vi "Autonomous Independent.vi"() -> ()   [LabVIEW 2019]
doc: "This VI is called when autonomous begins, and will automatically be terminated when autonomous ends. You can carry out timed or sensor driven robot movement independently without needing to return to the caller."
uses:
  <vilib>/Rock Robotics/WPI/ThirdParty/Phoenix-LabVIEW/Motor Controller/Controls/CTRE_Phoenix_MotorControl_ControlMode.ctl
  <vilib>/Rock Robotics/Network Tables/NT Read String.vi
  GlobalRefnum.vi
  Global Vars.vi
  <vilib>/Rock Robotics/WPI/ThirdParty/Phoenix-LabVIEW/Motor Controller/Get/CTRE_Phoenix_MotorController_GetSelectedSensorData.vi
  <vilib>/Rock Robotics/WPI/Utilities/WPI_GetSetVariantRefNum.vi
  Joystick_Buttons.vi
  <vilib>/Rock Robotics/Network Tables/NT Write Number.vi
  <vilib>/Rock Robotics/Network Tables/NT Write Numeric Array.vi
panel:
  in  "Travel Distance (In) 6":i32=223200
  out "Left Pos (In) 7":i32
  out "Right Pos (In) 7":i32
  in  "DriveK 7":dbl=0.01 min=0.0 max=1.0 step=0.05
  in  "MaxDrive Fast 5":dbl(slide)=0.7518248175182481 min=0.0 max=1.0 step=0.01 scale=0.0..1.0
  in  "DriveDeadband 7":dbl=100.0
  in  "MaxDrive Slow 4":dbl(slide)=0.49635036496350365 min=0.0 max=1.0 step=0.01 scale=0.0..1.0
  out "Left Pos (In) 6":i32
  out "Right Pos (In) 6":i32
  in  "DriveK 6":dbl=0.01 min=0.0 max=1.0 step=0.05
  in  "MaxDrive Fast 4":dbl(slide)=0.7518248175182481 min=0.0 max=1.0 step=0.01 scale=0.0..1.0
  in  "DriveDeadband 6":dbl=100.0
  in  "MaxDrive Slow 3":dbl(slide)=0.49635036496350365 min=0.0 max=1.0 step=0.01 scale=0.0..1.0
  in  "Reverse? 6":bool=TRUE
  in  "Tab Control":T1(tab)
  in  "Travel Distance (In)":dbl=36.0
  out "Left Pos (In)":dbl
  out "Right Pos (In)":dbl
  in  "Reverse?":bool
  in  "Output":dbl(slide)=-0.5 scale=0.0..1.0
  in  "Travel Distance (In) 3":i32=30000
  in  "Reverse? 3":bool
  out "Left Pos (In) 3":i32
  out "Right Pos (In) 3":i32
  in  "DriveK 2":dbl=0.01 min=0.0 max=1.0 step=0.05
  in  "DriveDeadband 2":dbl=100.0
  in  "MaxDrive 2":dbl(slide)=0.6824817518248175 min=0.0 max=1.0 step=0.01 scale=0.0..1.0
  in  "Reverse? 4":bool=TRUE
  out "Right Pos (In) 4":i32
  out "Left Pos (In) 4":i32
  in  "Travel Distance (In) 4":i32=223200
  in  "DriveDeadband 3":dbl=100.0
  in  "DriveK 3":dbl=0.01 min=0.0 max=1.0 step=0.05
  in  "MaxDrive Fast":dbl(slide)=0.7518248175182481 min=0.0 max=1.0 step=0.01 scale=0.0..1.0
  in  "MaxDrive Slow":dbl(slide)=0.49635036496350365 min=0.0 max=1.0 step=0.01 scale=0.0..1.0
  in  "DriveDeadband 4":dbl=100.0
  in  "DriveDeadband 5":dbl=100.0
  out "Right Pos (In) 5":i32
  out "Left Pos (In) 5":i32
  in  "DriveK 4":dbl=0.01 min=0.0 max=1.0 step=0.05
  in  "DriveK 5":dbl=0.01 min=0.0 max=1.0 step=0.05
  in  "Reverse? 5":bool=TRUE
  in  "Travel Distance (In) 5":i32=190000
  in  "MaxDrive Slow 2":dbl(slide)=0.5072992700729927 min=0.0 max=1.0 step=0.01 scale=0.0..1.0
  in  "MaxDrive Fast 2":dbl(slide)=0.5072992700729927 min=0.0 max=1.0 step=0.01 scale=0.0..1.0
  in  "MaxDrive Fast 3":dbl(slide)=0.5072992700729927 min=0.0 max=1.0 step=0.01 scale=0.0..1.0
  in  "Travel Distance 2":i32=190000
  out "Right Pos (In) 2":i32
  out "Left Pos (In) 2":i32
  in  "Travel Distance (In) 2":i32=18474
  in  "Reverse? 2":bool
  in  "DriveK":dbl=0.01 min=0.0 max=1.0 step=0.05
  in  "MaxDrive":dbl(slide)=0.6824817518248175 min=0.0 max=1.0 step=0.01 scale=0.0..1.0
  in  "DriveDeadband":dbl=100.0
  out "Current Movement, for debugging":T2 {"Y Joystick Value" scale=1.0..-1.0; "X Joystick Value" scale=-1.0..1.0}
  in  "Array of robot movements":T3(array[cluster])=[{"X Joystick Value"=0.39393939393939403, "Y Joystick Value"=0.0, "Delay (sec)"=1.0, "Movement Name"="turn"}, {"X Joystick Value"=-0.3737373737373737, "Y Joystick Value"=0.0, "Delay (sec)"=1.0, "Movement Name"="turn back"}] {"Y Joystick Value" scale=1.0..-1.0; "X Joystick Value" scale=-1.0..1.0}
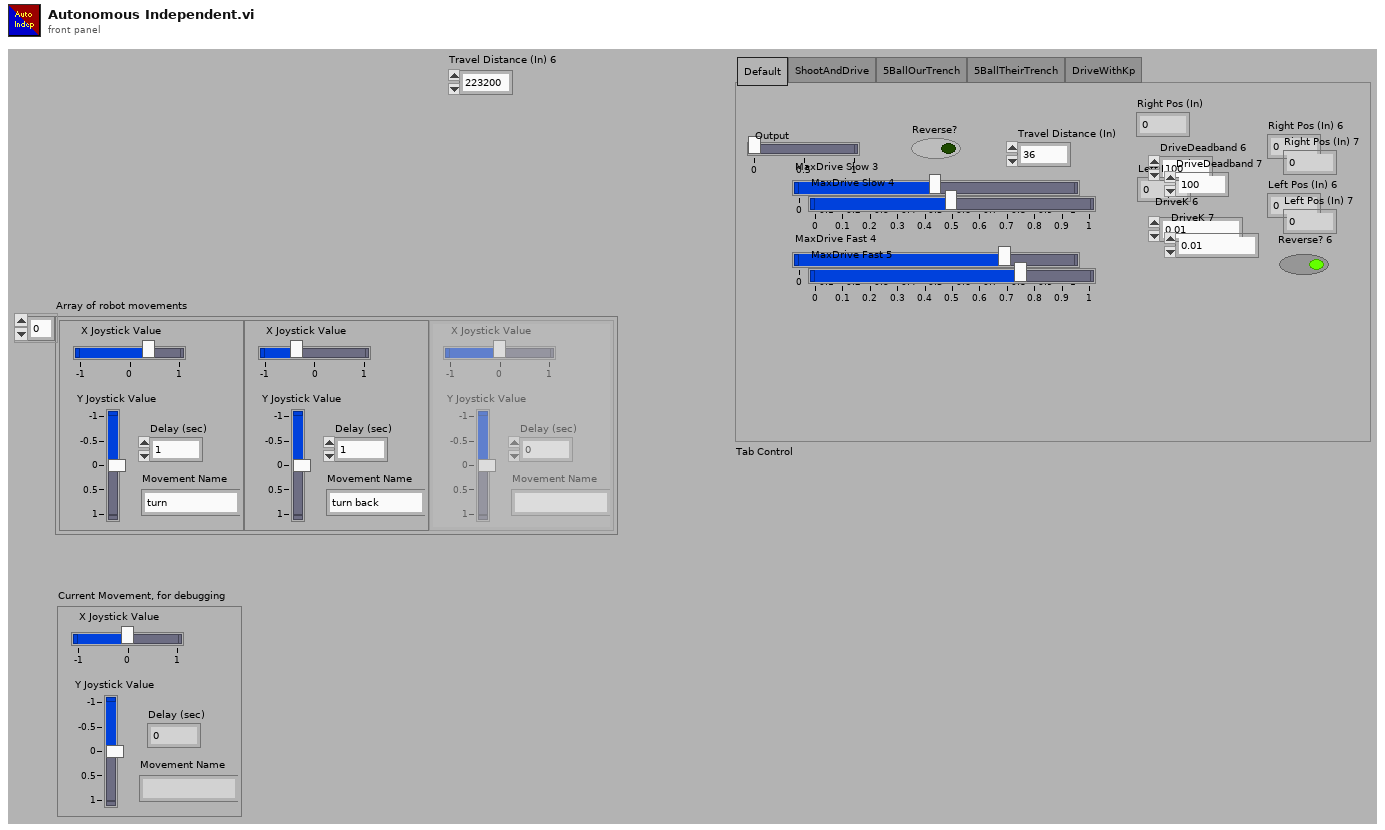
[diagram p1: front panel]
types:
  T1 = enum32{"Default", "ShootAndDrive", "5BallOurTrench", "5BallTheirTrench", "DriveWithKp"}
  T2 = cluster{"X Joystick Value":dbl, "Y Joystick Value":dbl, "Delay (sec)":dbl, "Movement Name":string}
  T3 = cluster{"X Joystick Value":dbl, "Y Joystick Value":dbl, "Delay (sec)":dbl, "Movement Name":string}[]
  T4 = typedef "WPI_JoystickDevRef.ctl" = cluster{"Device":T5}
  T5 = typedef "WPI_JoystickDeviceEnum.ctl" = enum16{"USB 0", "USB 1", "USB 2", "USB 3", "USB 4", "USB 5"}
  T6 = enum16{"Pause1", "Aim", "Drive", "End", "Init", "Shoot"}
  T7 = enum16{"Pause3", "Pause2", "Shoot2", "Aim2", "Drive2", "Pause1", "Aim", "Drive", "End", "Init", "Shoot"}
  T8 = enum16{"Drive2", "Aim2", "Pause2", "Pause1", "Aim", "Drive", "End", "Init", "Shoot"}
  T9 = typedef "WPI_MotorControlDeviceRef.ctl" = cluster{"DeviceStatus":errorcluster, "Type":T10, "PWM":cluster{"PWM Channel":T11, "DeadBand":T12}, "CAN":cluster{"Device Number":u8, "SetOutput VI Ref":variant, "GetOutput VI Ref":variant, "Enable VI Ref":variant, "Disable VI Ref":variant, "Data":variant}, "Invert":bool, "DIO PWM":cluster{"PWM \"Enable\" Channel":T11, "DIOChannel":T13, "PWM Rate":dbl}}
  T10 = typedef "WPI_MotorControlType.ctl" = enum16{"PWM", "CAN", "DIO PWM"}
  T11 = typedef "FPGA_DIOPWMChannel.ctl" = enum8{"PWM 0", "PWM 1", "PWM 2", "PWM 3", "PWM 4", "PWM 5", "PWM 6", "PWM 7", "PWM 8", "PWM 9", "PWM MXP 0", "PWM MXP 1", "PWM MXP 2", "PWM MXP 3", "PWM MXP 4", "PWM MXP 5", "PWM MXP 6", "PWM MXP 7", "PWM MXP 8", "PWM MXP 9", "Invalid"}
  T12 = typedef "WPI_PWMDeadband.ctl" = cluster{"Name":string, "maxPositivePwm":i32, "minPositivePwm":i32, "centerPwm":i32, "maxNegativePwm":i32, "minNegativePwm":i32, "angularRange":u16}
  T13 = typedef "FPGA_DIOChannel.ctl" = enum8{"DIO 0", "DIO 1", "DIO 2", "DIO 3", "DIO 4", "DIO 5", "DIO 6", "DIO 7", "DIO 8", "DIO 9", "DIO MXP 0", "DIO MXP 1", "DIO MXP 2", "DIO MXP 3", "DIO MXP 4", "DIO MXP 5", "DIO MXP 6", "DIO MXP 7", "DIO MXP 8", "DIO MXP 9", "DIO MXP 10", "DIO MXP 11", "DIO MXP 12", "DIO MXP 13", "DIO MXP 14", "DIO MXP 15", "SPI Port CS1", "SPI Port CS2", "SPI Port CS3", "SPI Port MISO", "SPI Port MOSI", "Invalid"}
  T14 = typedef "CTRE_Phoenix_MotorControl_ControlMode.ctl" = u16
  T15 = typedef "WPI_RobotDriveDevRef.ctl" = cluster{"DevStatus":errorcluster, "Motors[]":T9[], "Square Inputs":bool, "Max Output":dbl}
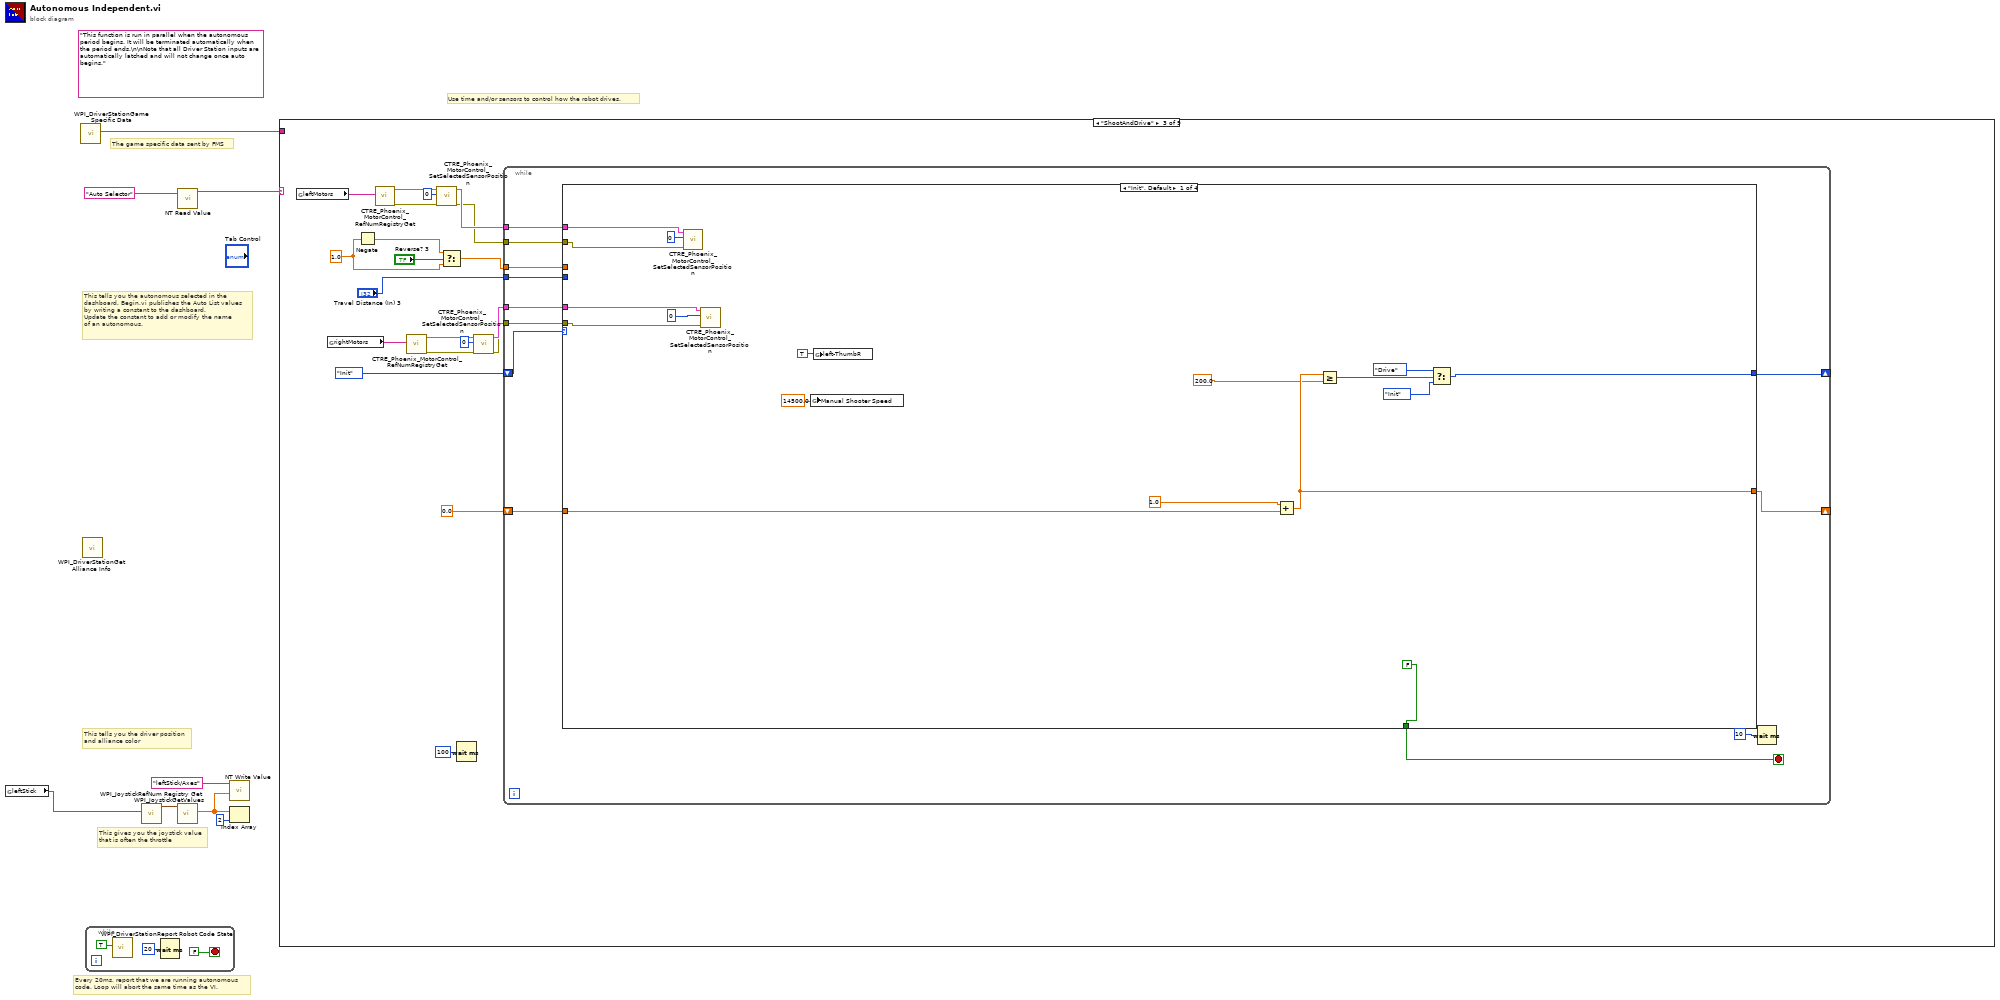
[diagram p0: block diagram]
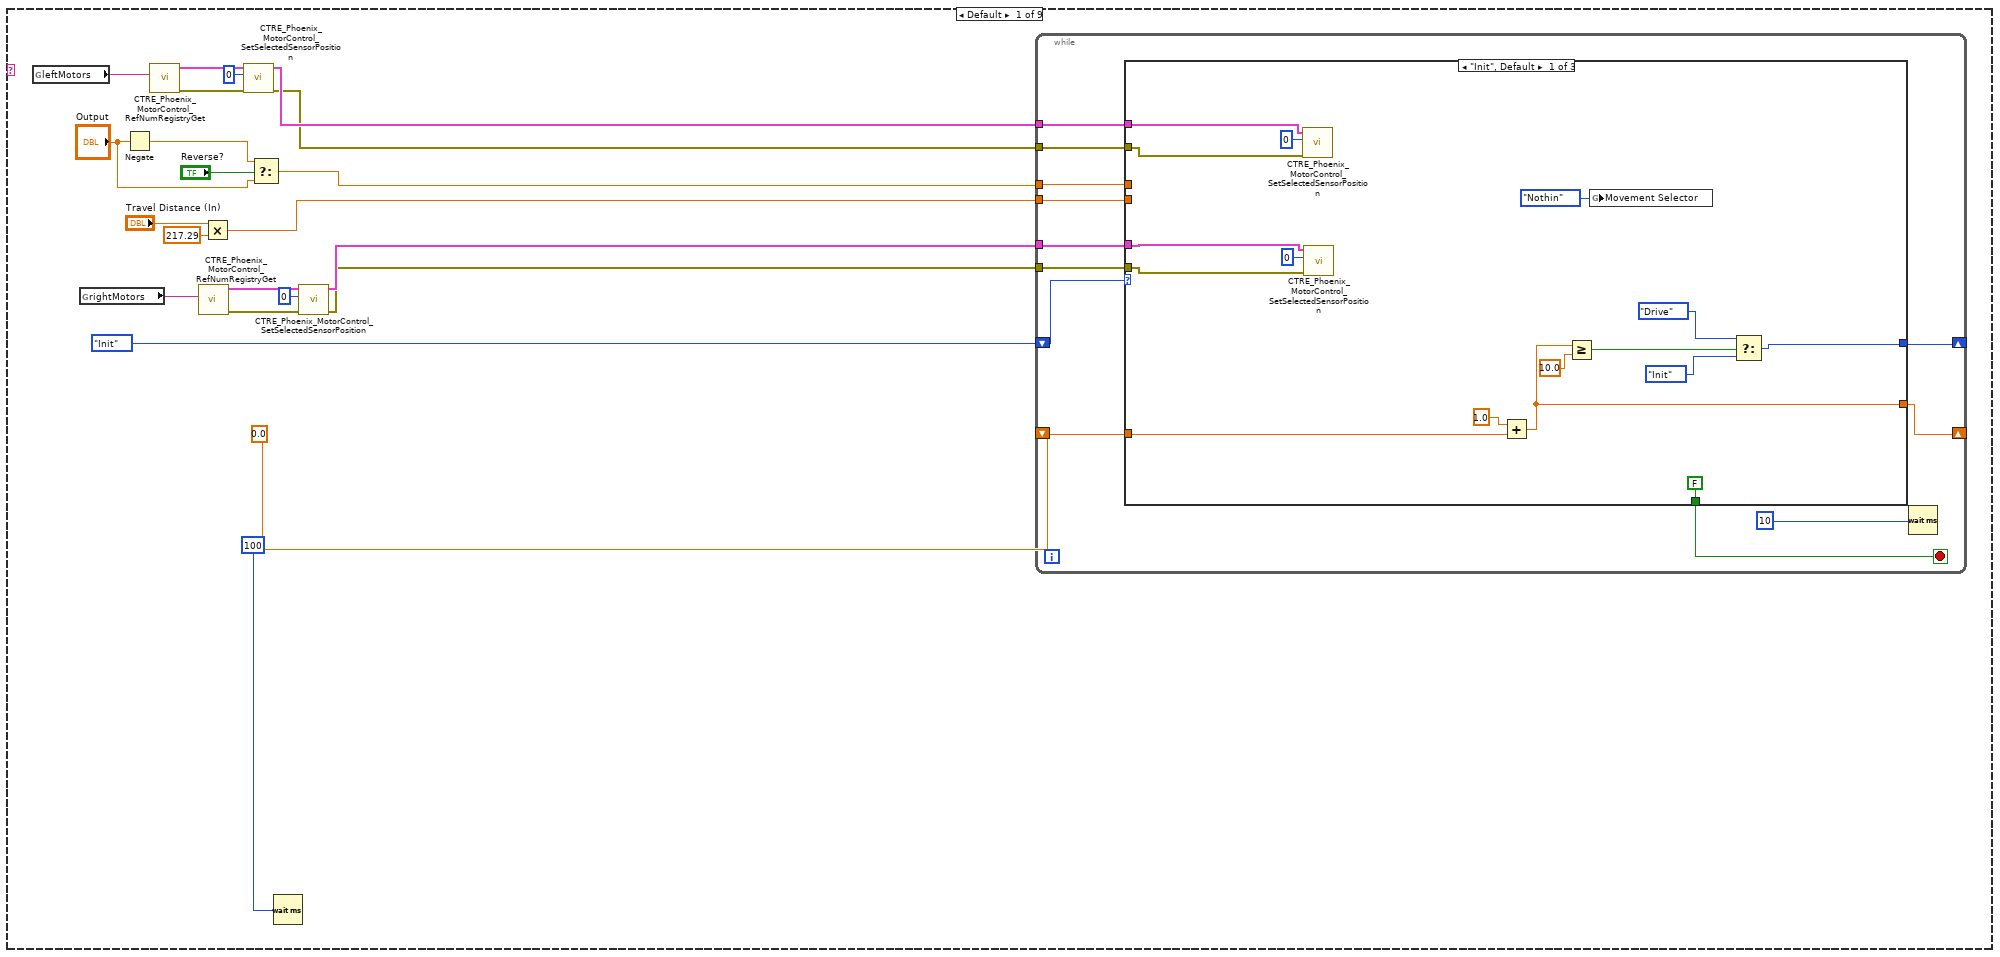
[diagram p2: hidden frame]
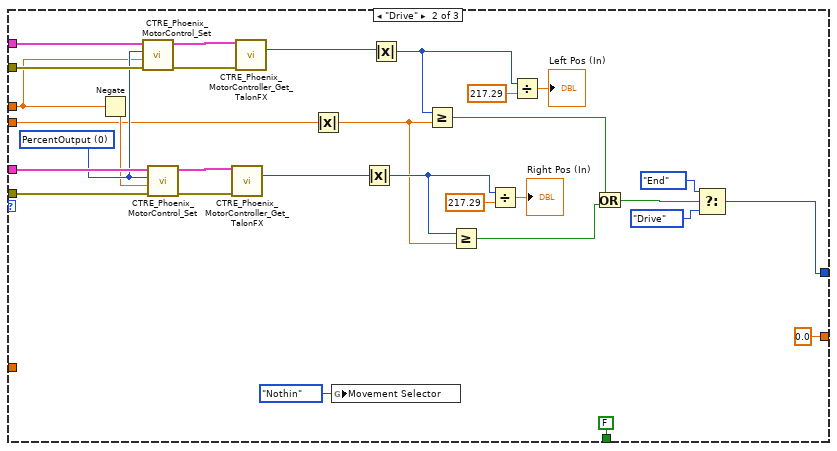
[diagram p3: hidden frame]
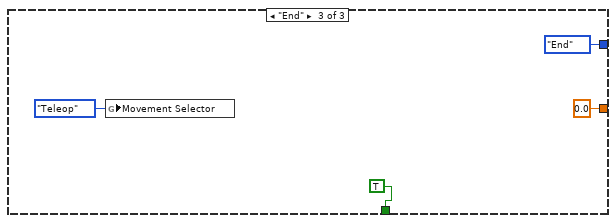
[diagram p4: hidden frame]
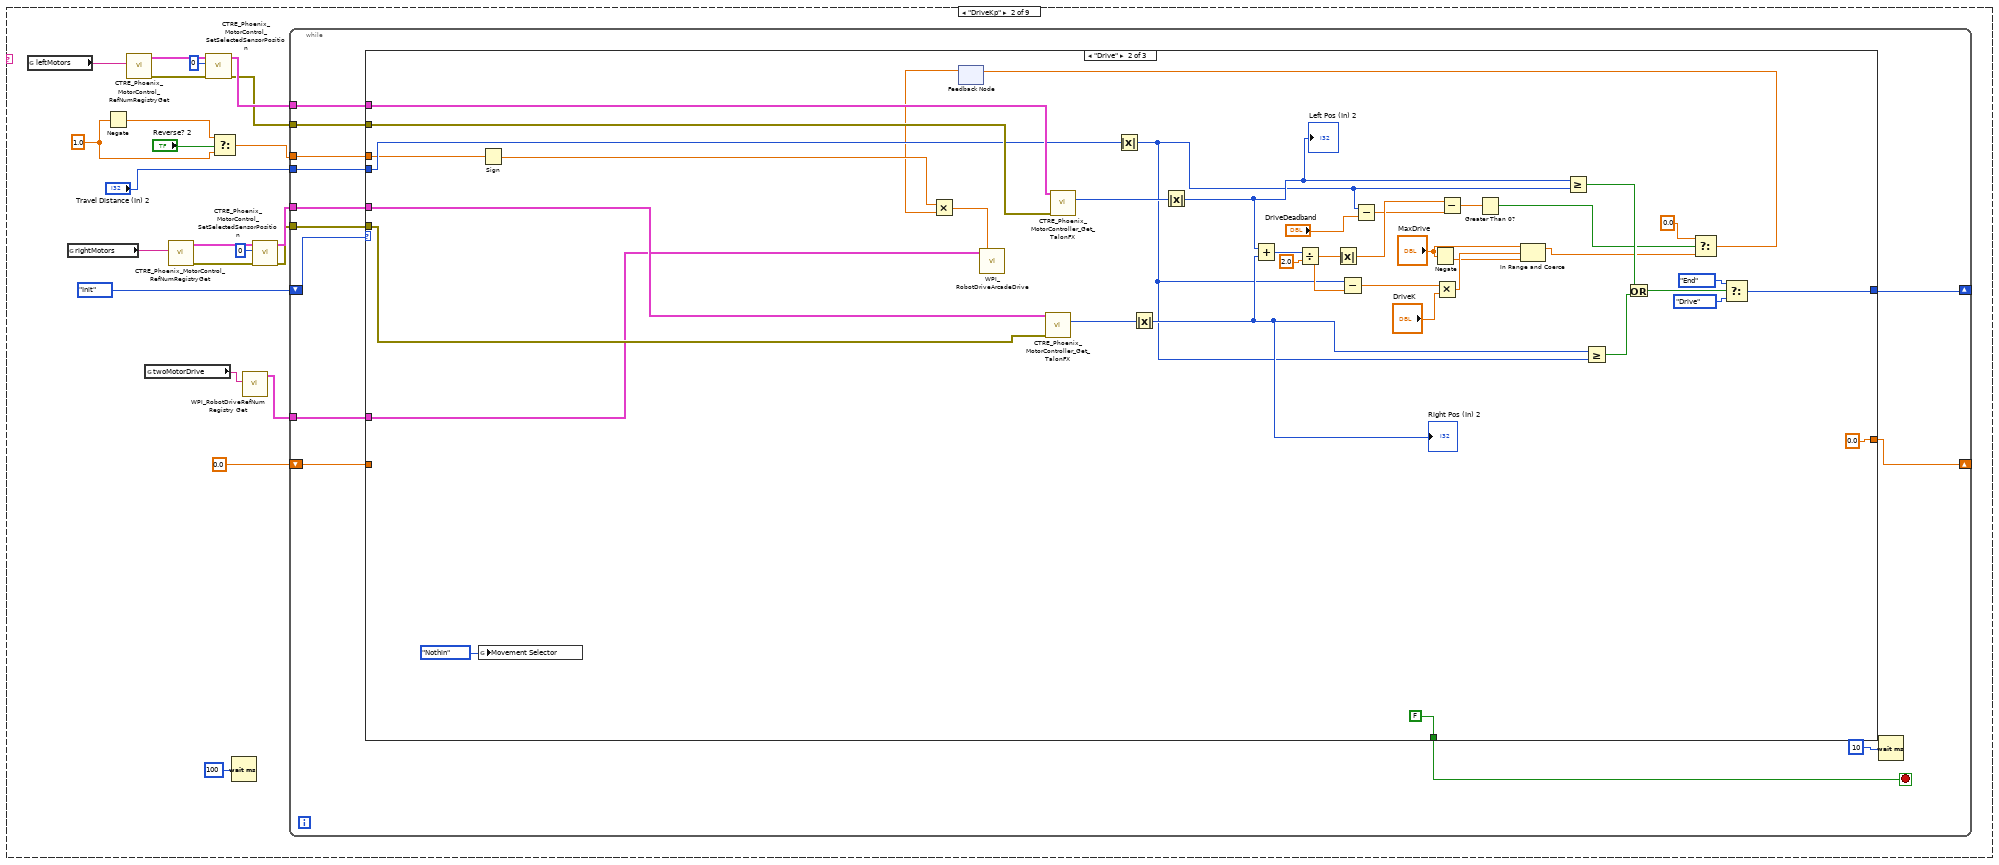
[diagram p5: hidden frame]
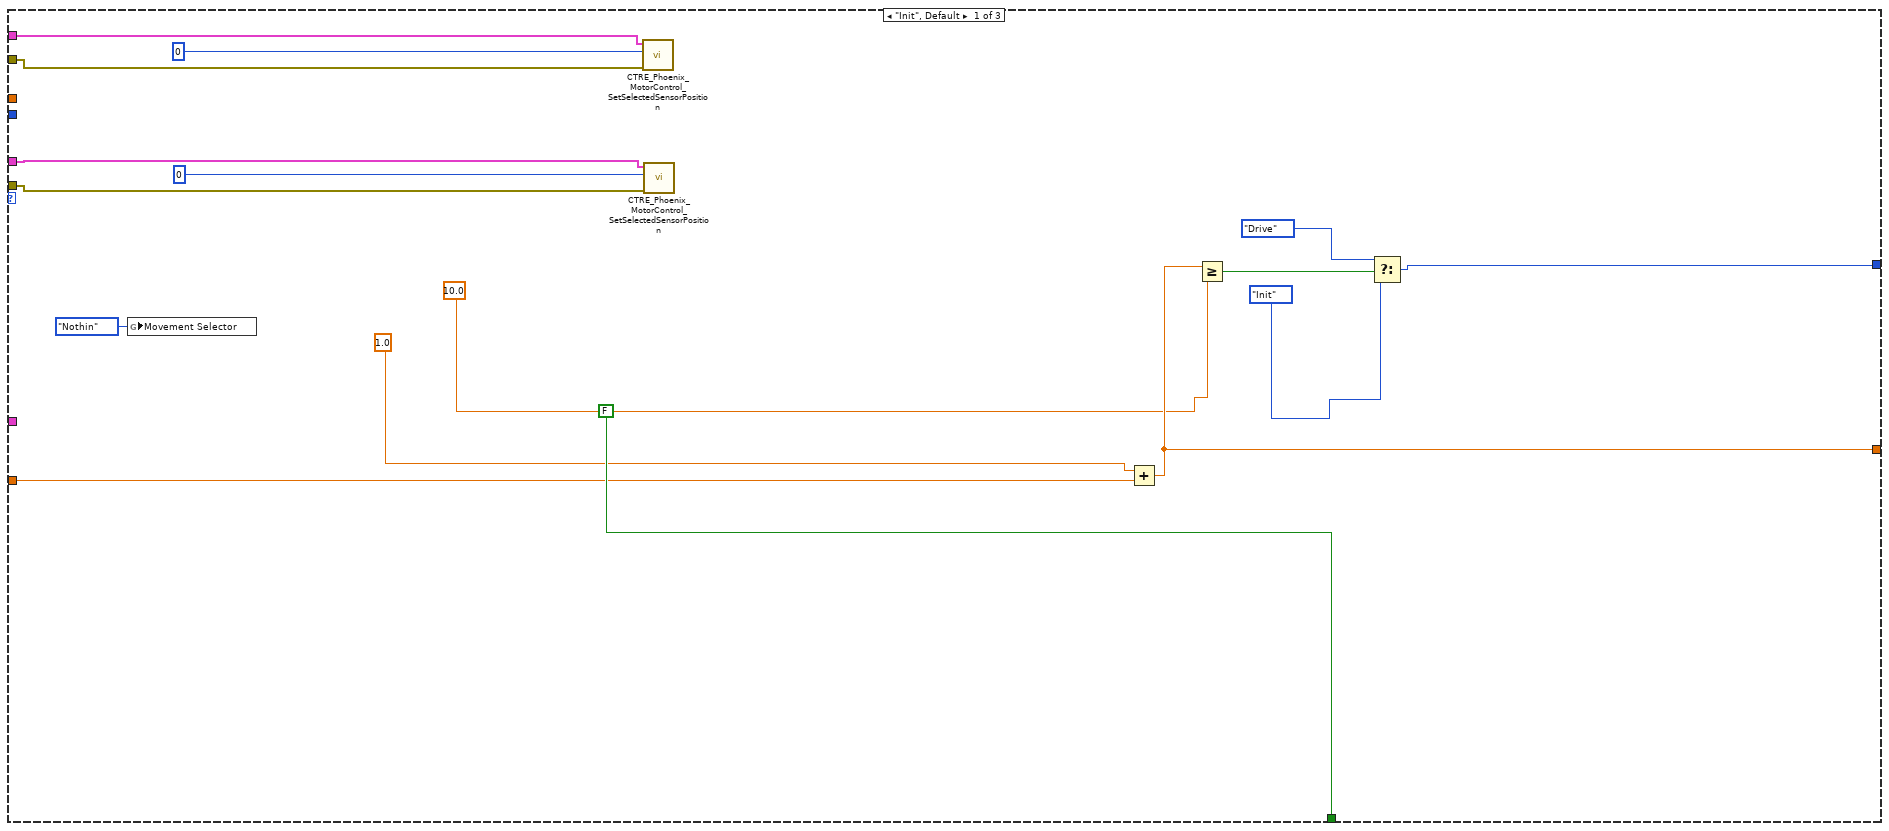
[diagram p6: hidden frame]
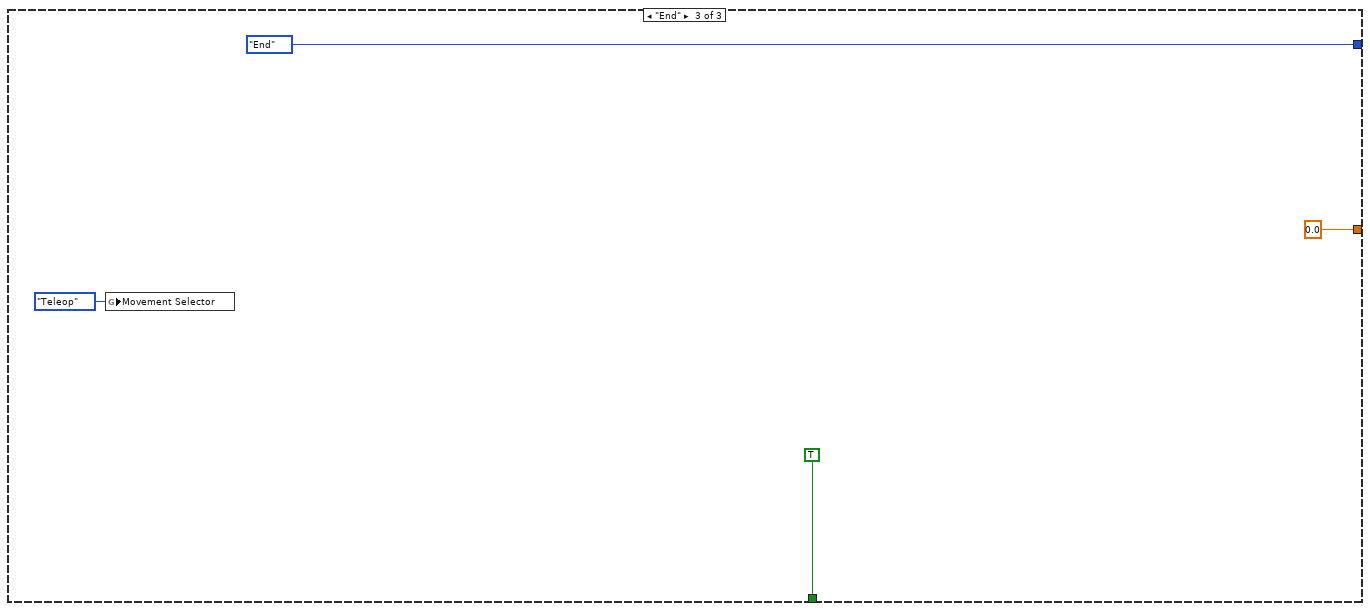
[diagram p7: hidden frame]
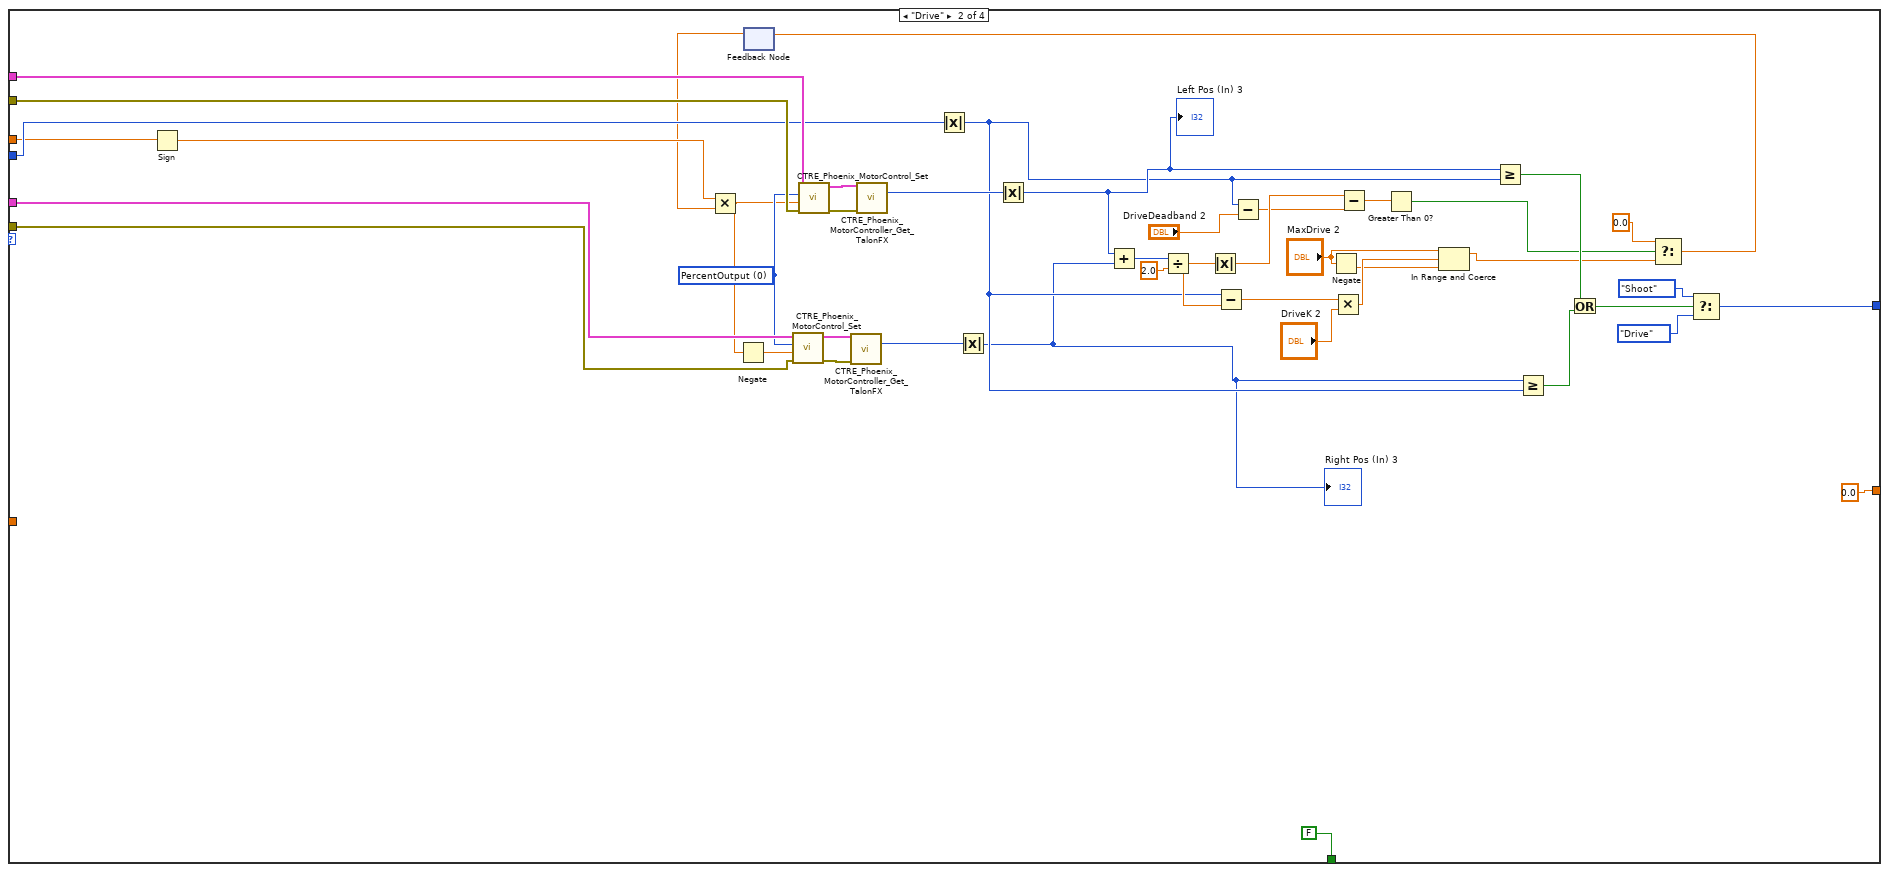
[diagram p8: hidden frame]
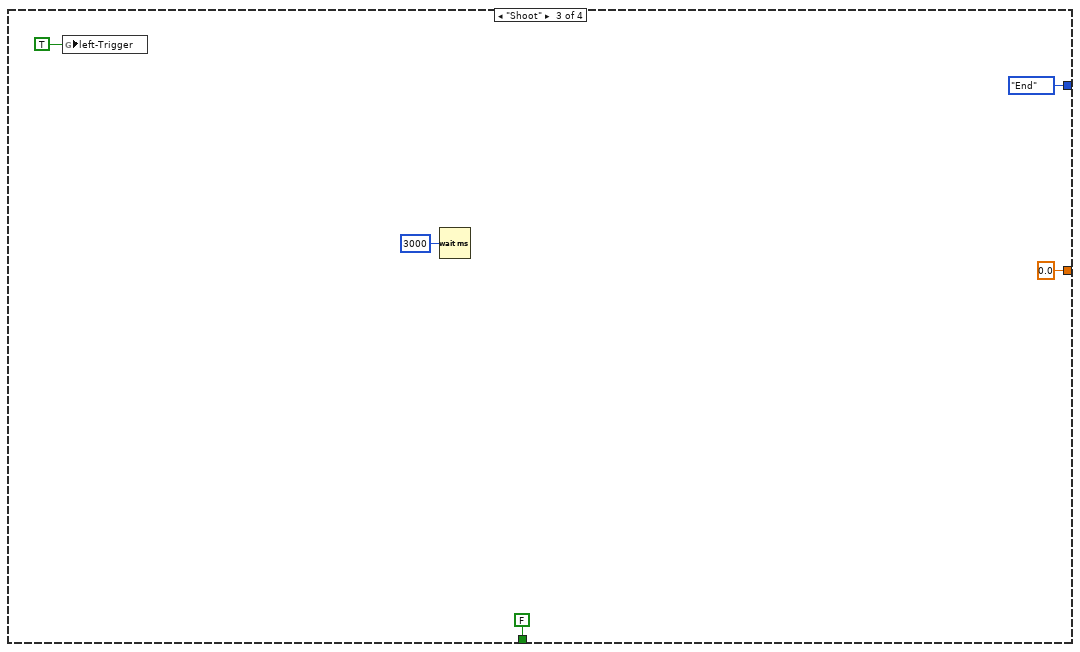
[diagram p9: hidden frame]
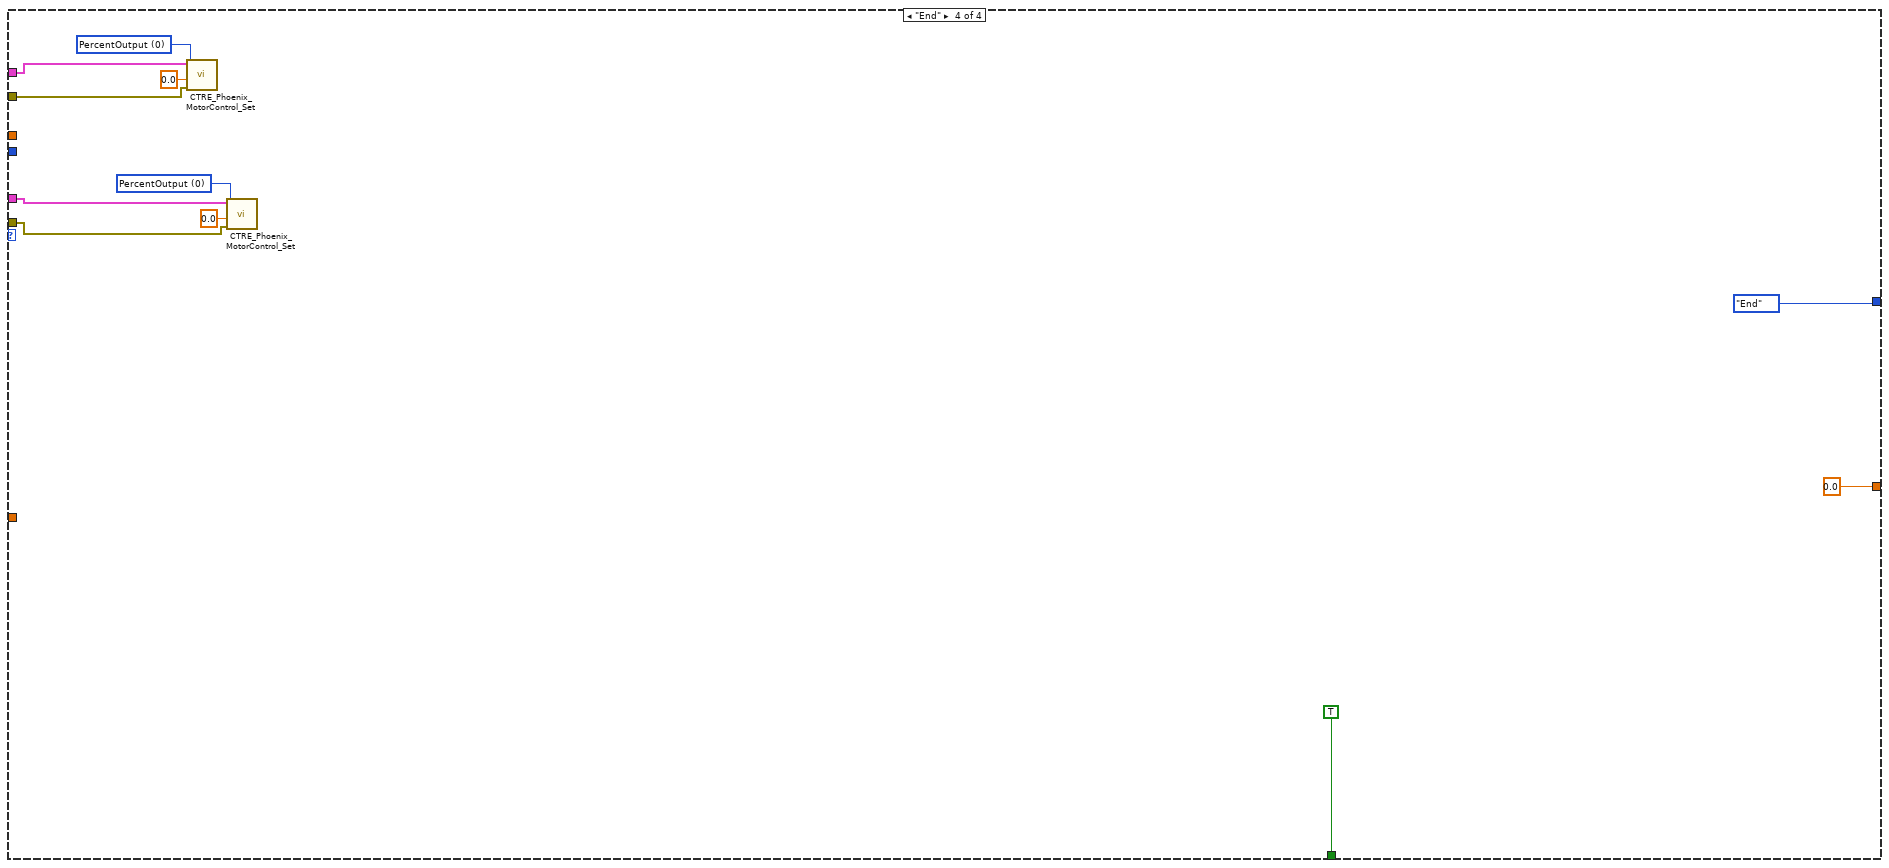
[diagram p10: hidden frame]
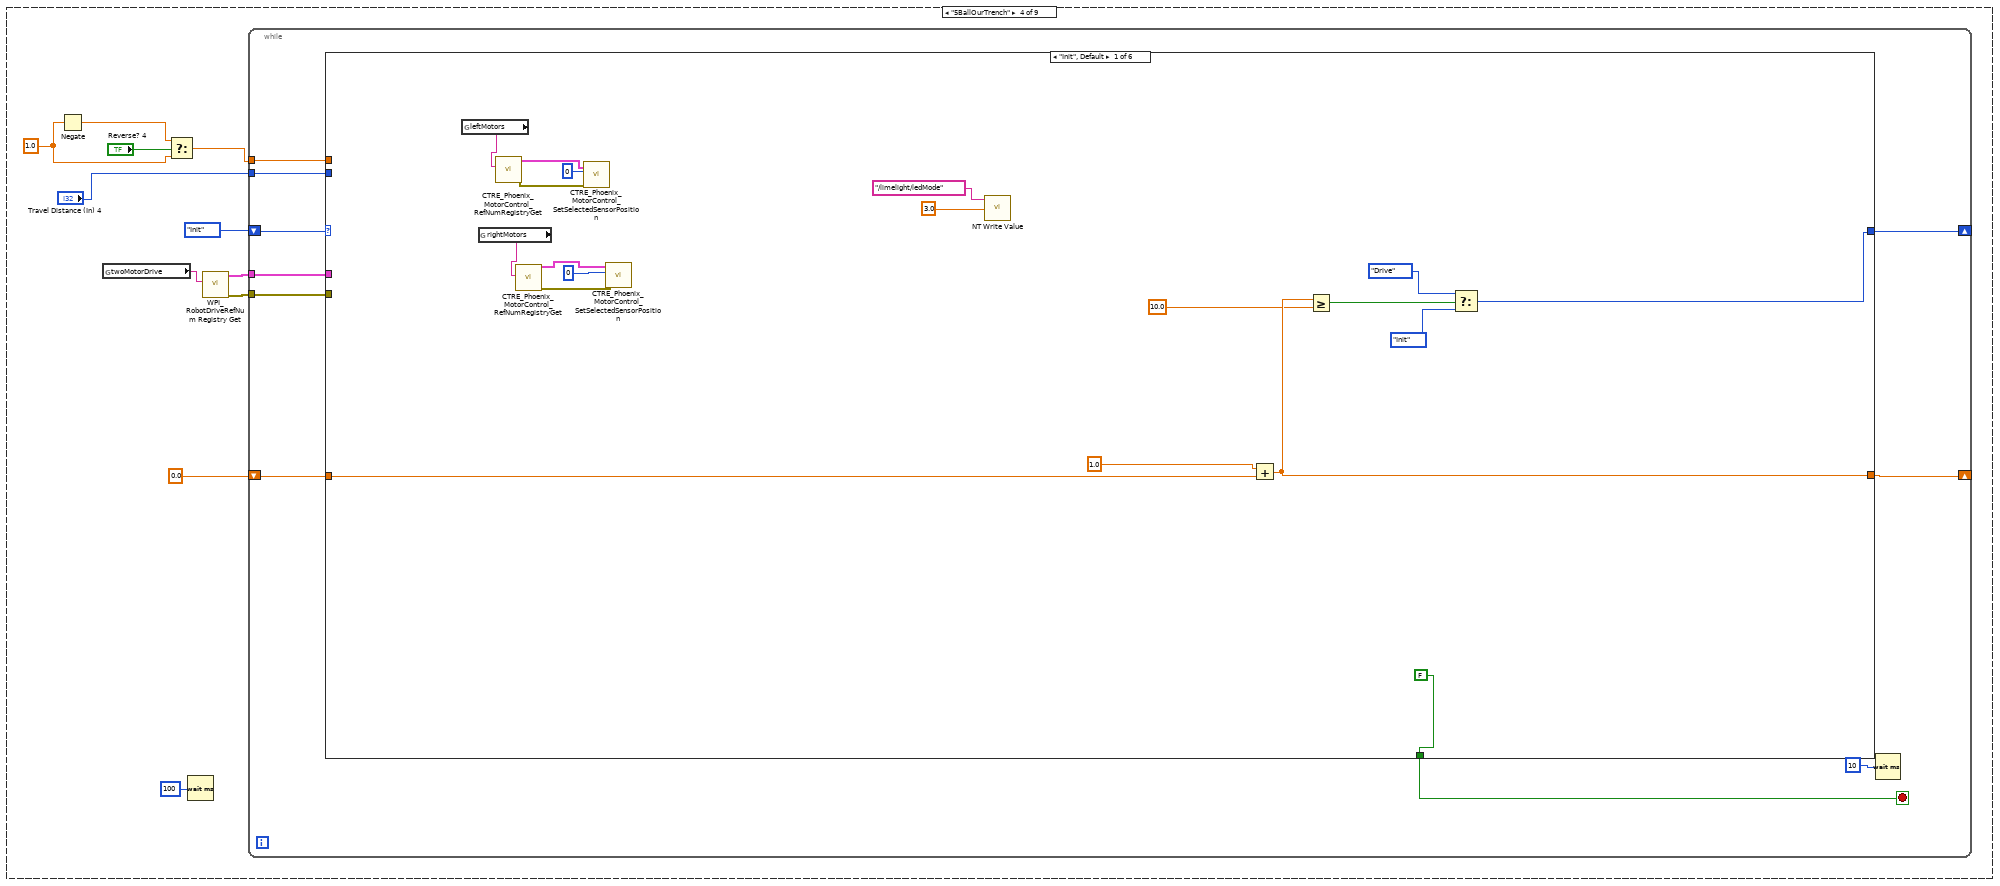
[diagram p11: hidden frame]
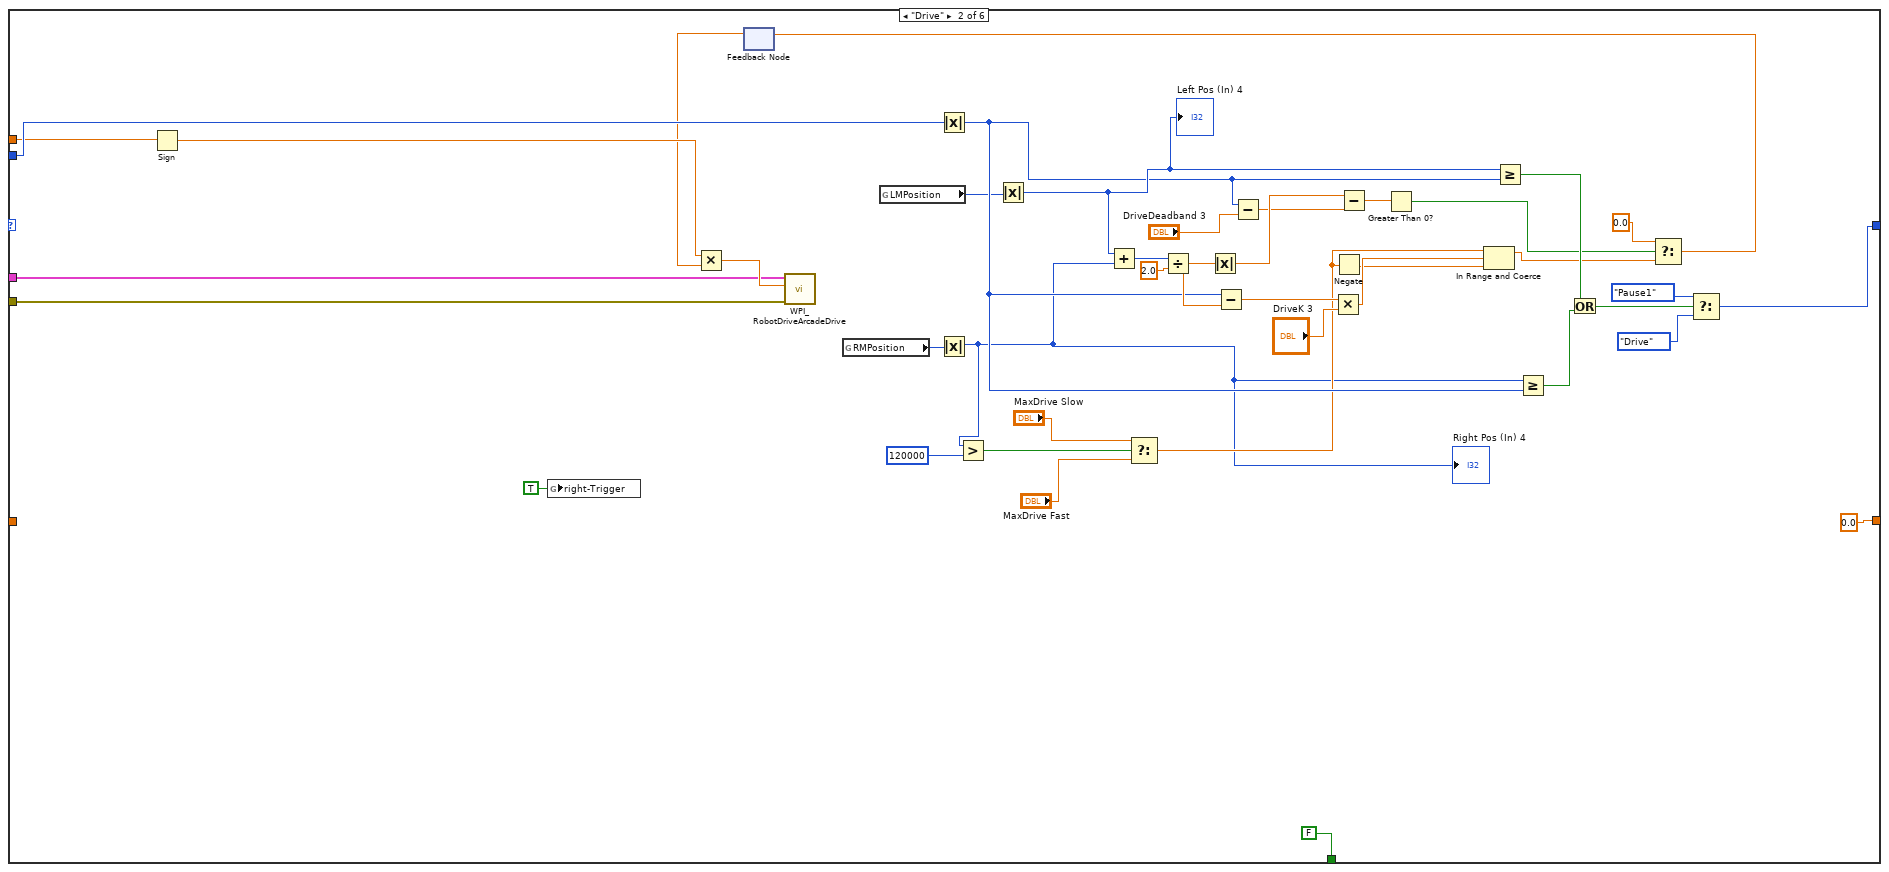
[diagram p12: hidden frame]
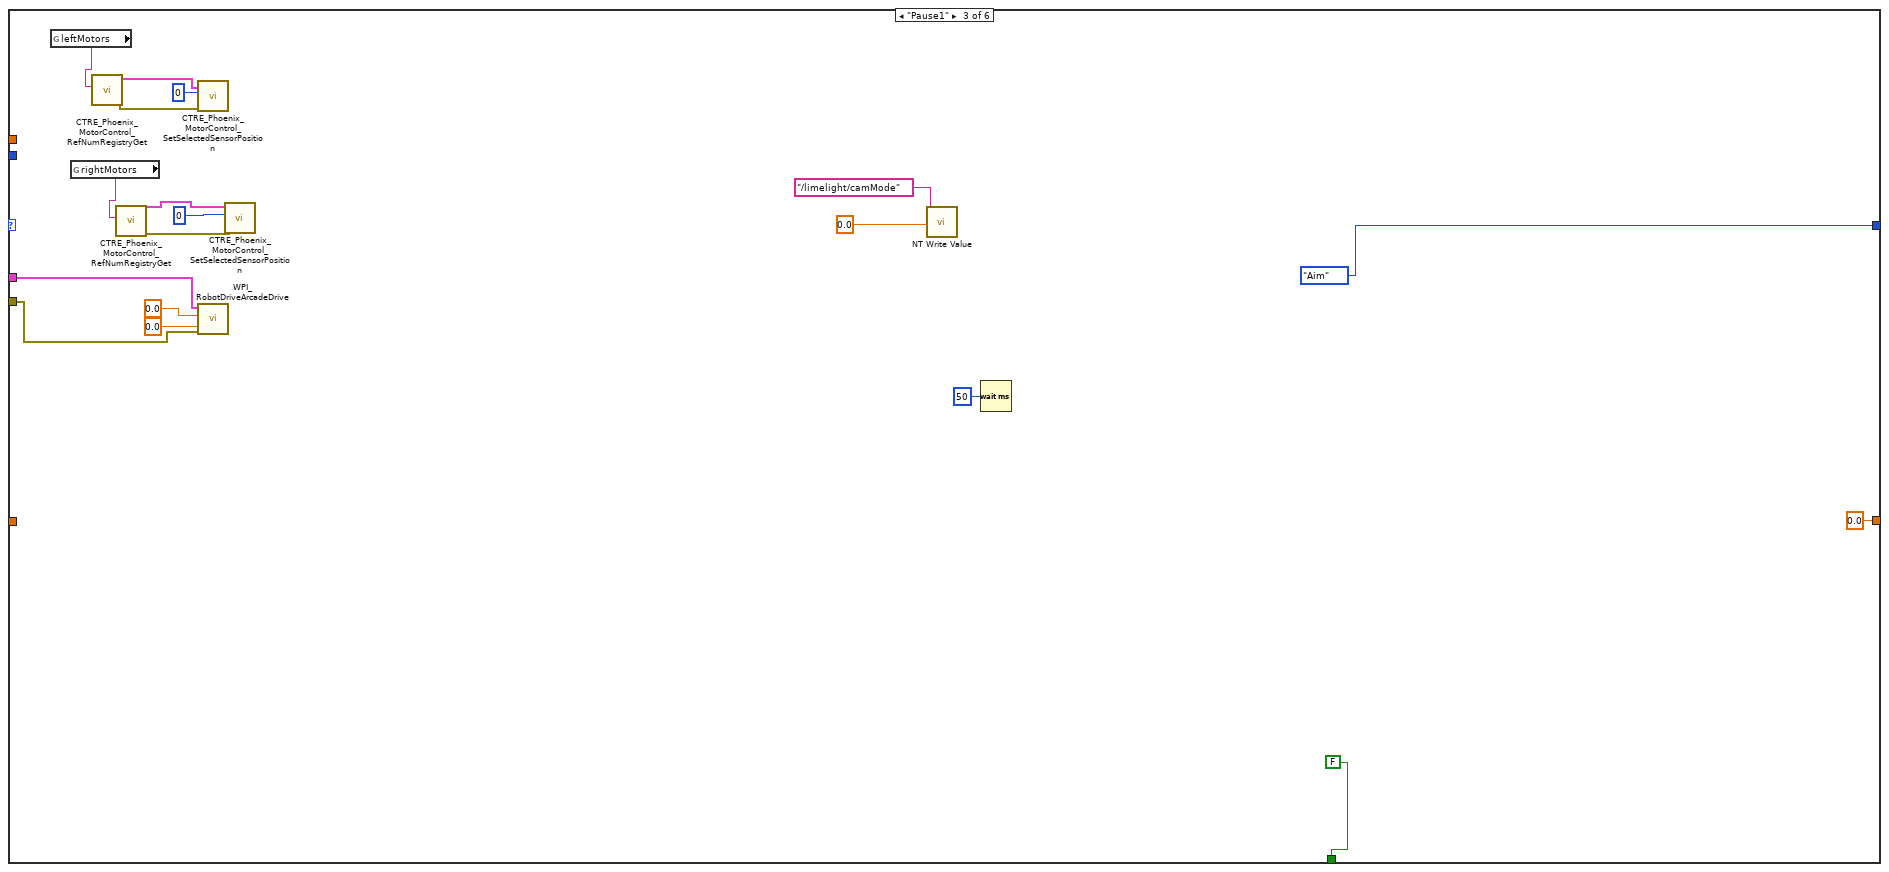
[diagram p13: hidden frame]
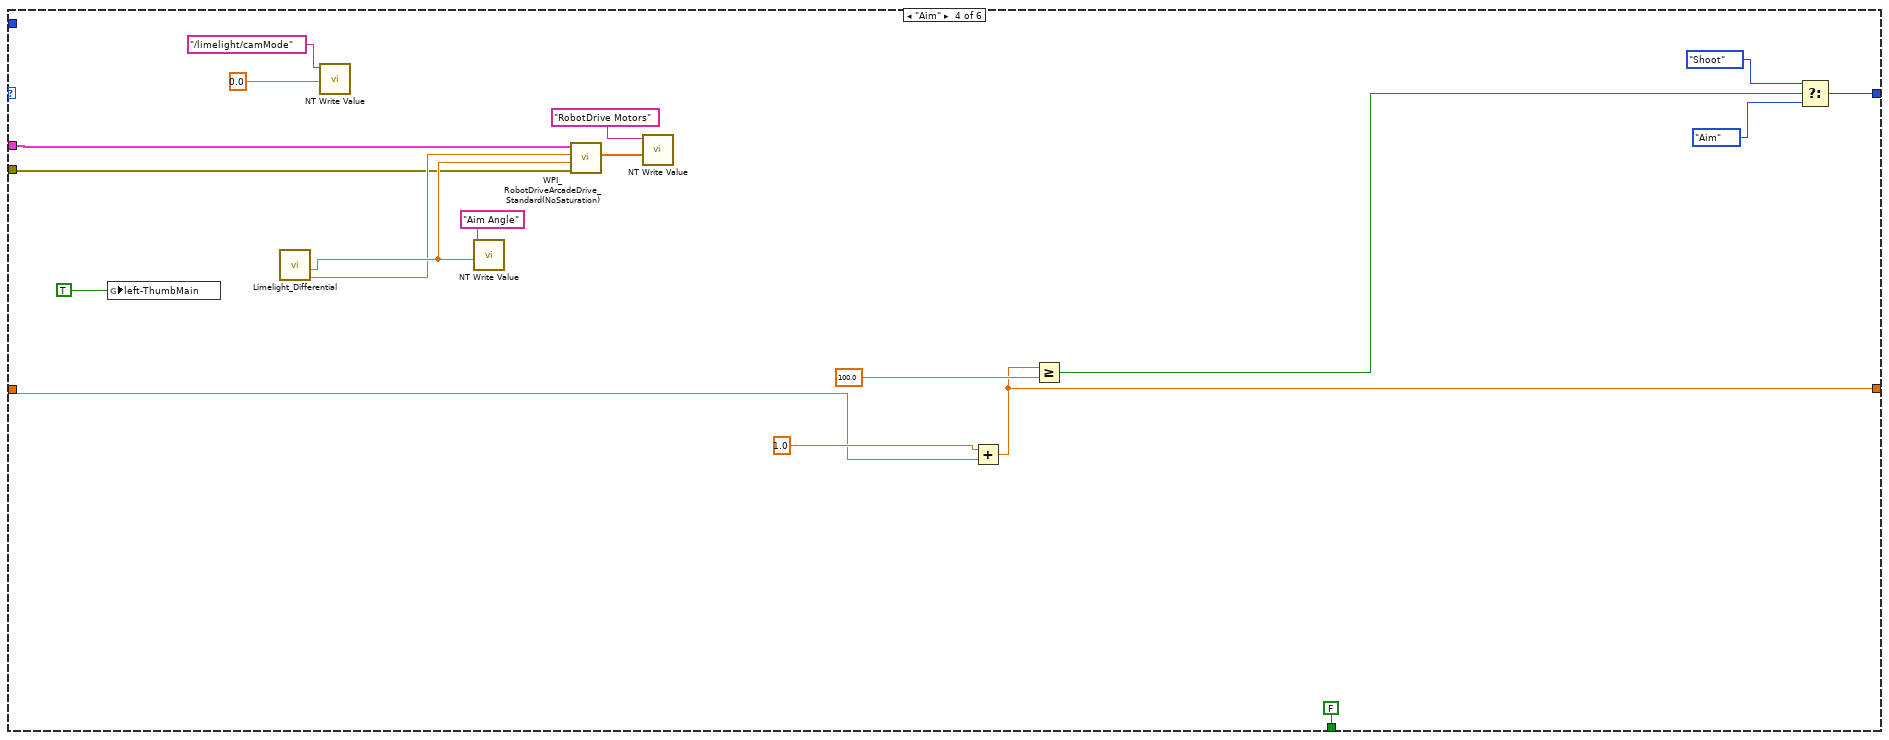
[diagram p14: hidden frame]
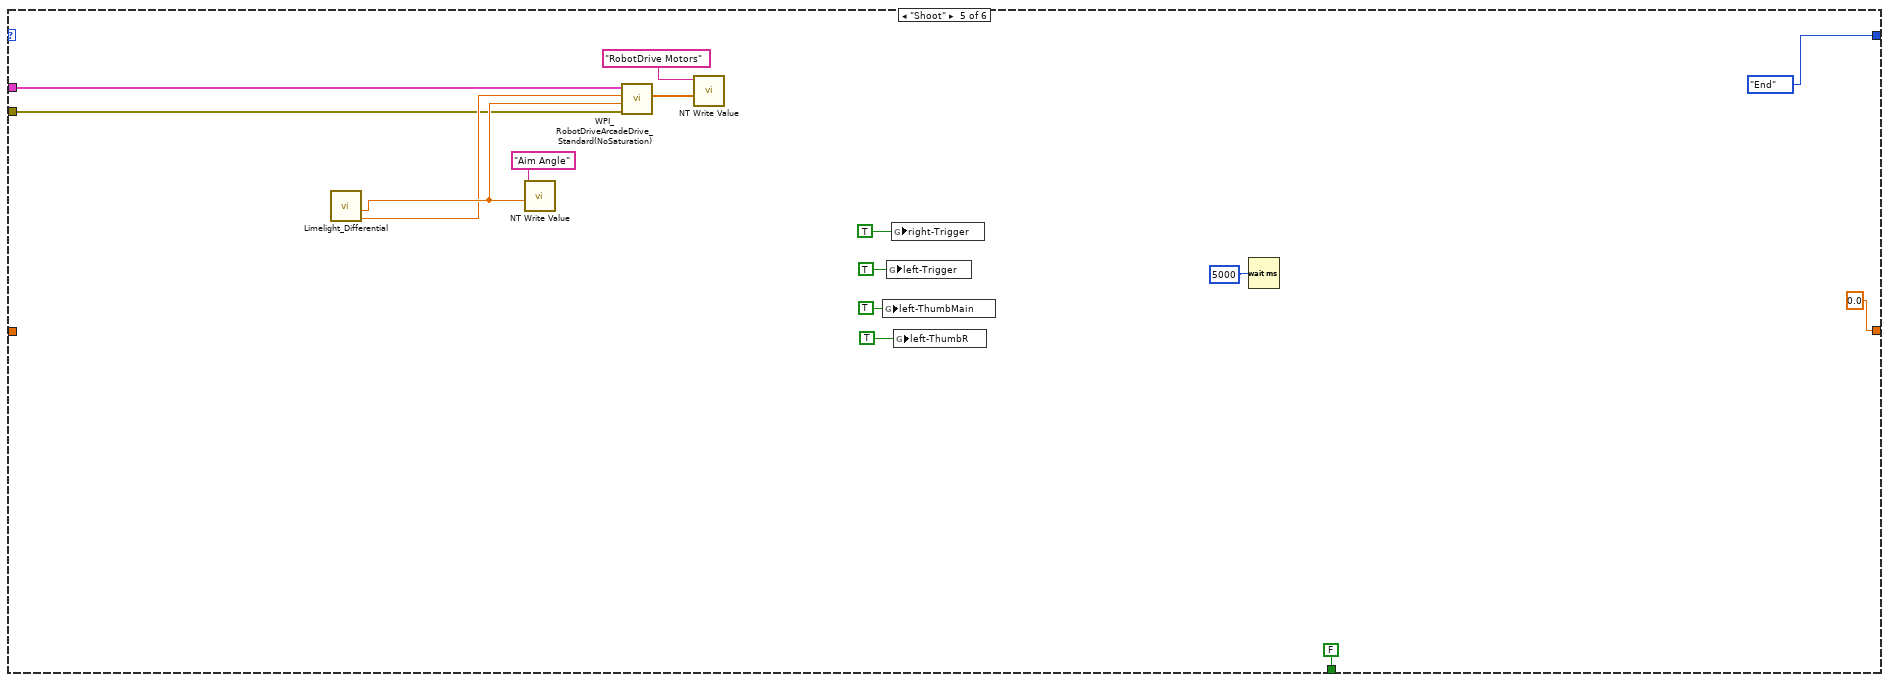
[diagram p15: hidden frame]
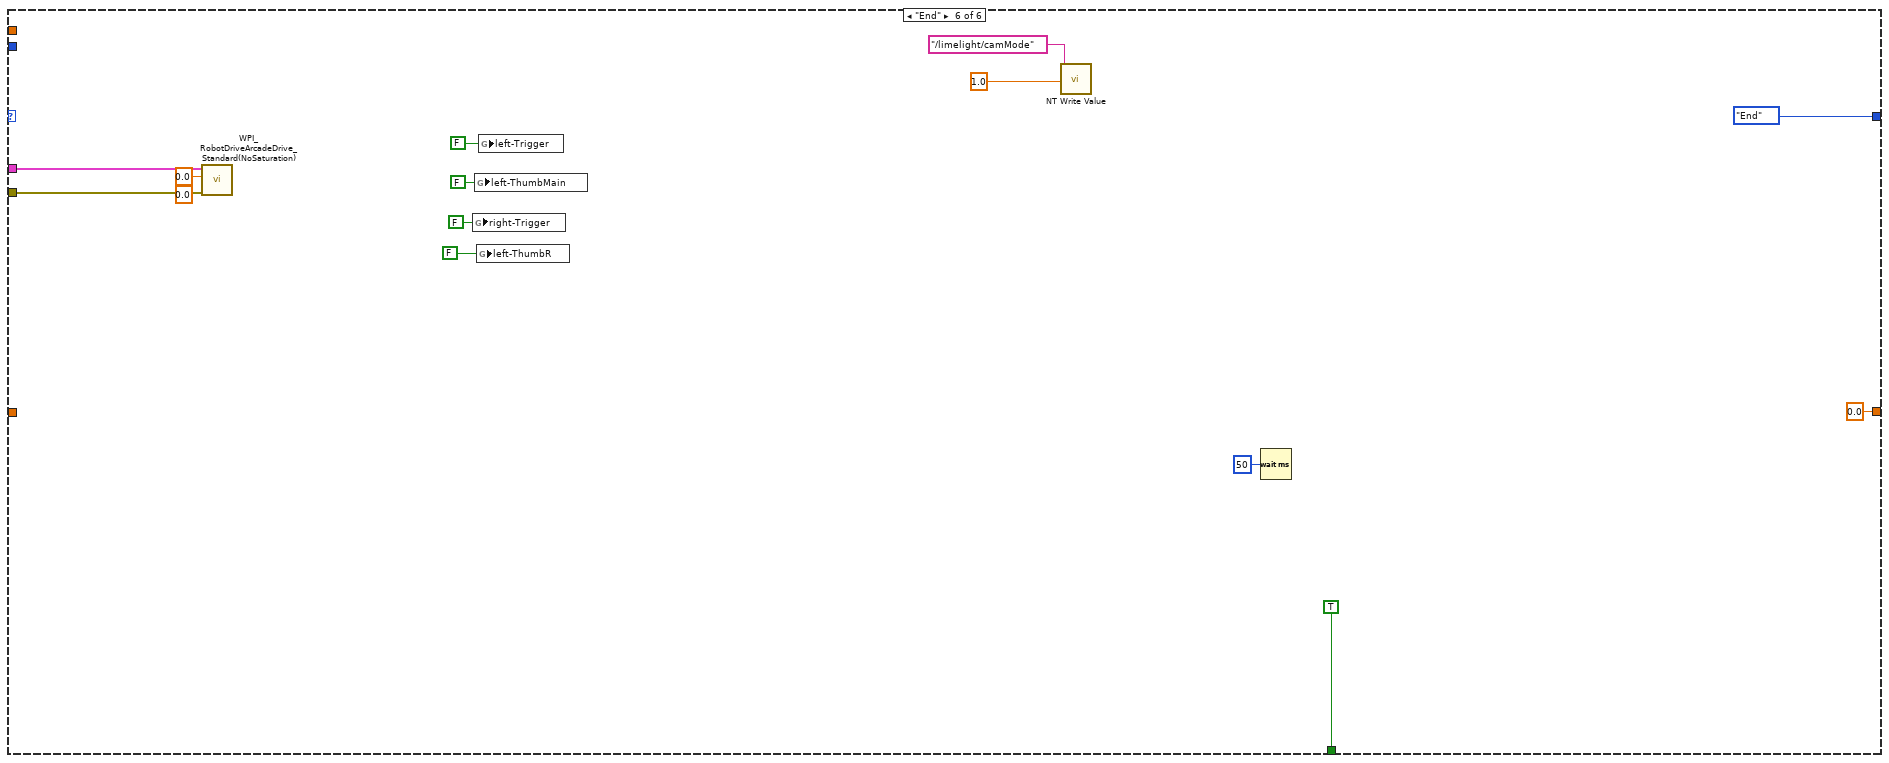
[diagram p16: hidden frame]
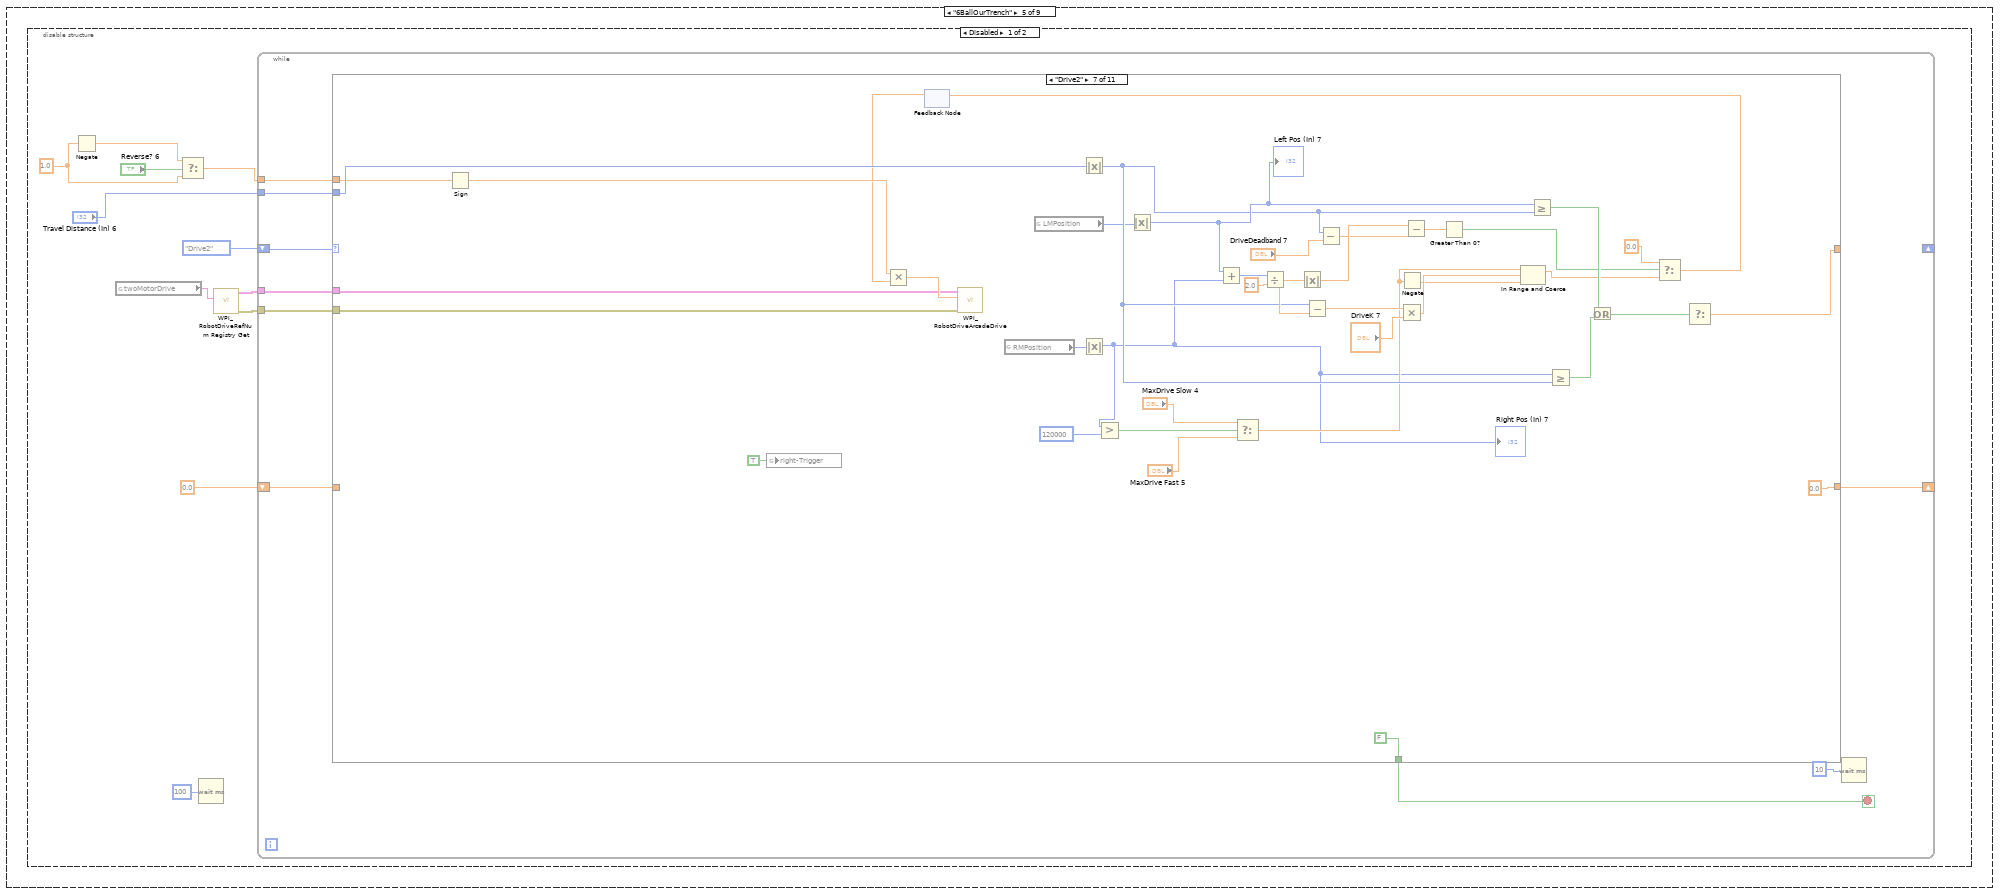
[diagram p17: hidden frame]
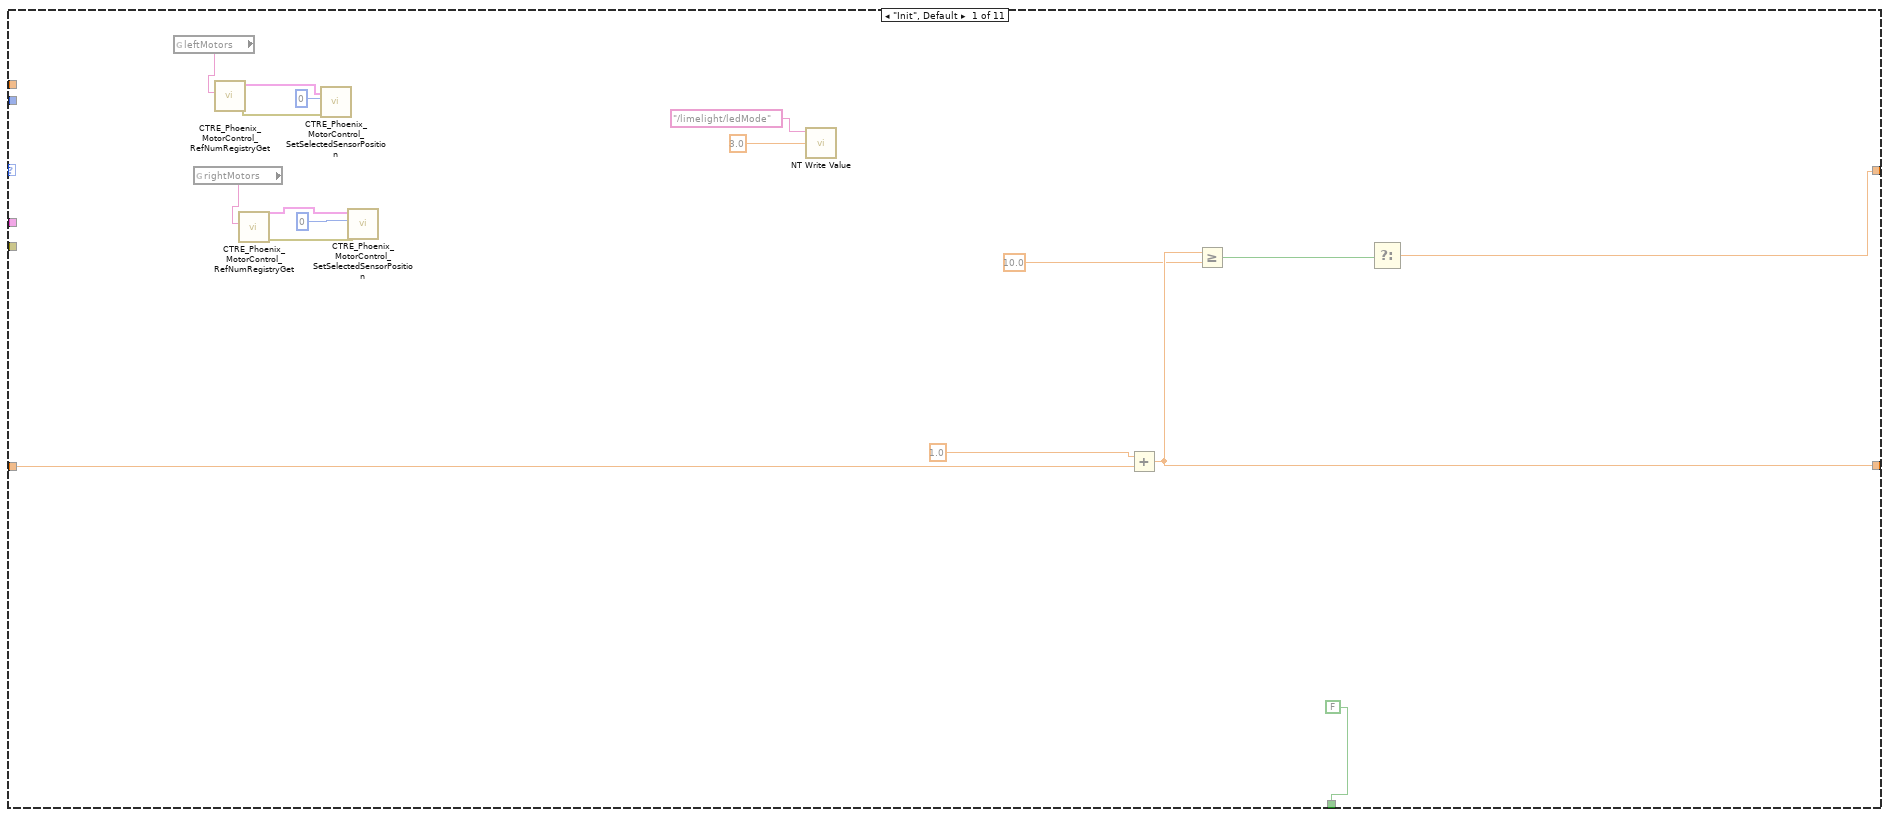
[diagram p18: hidden frame]
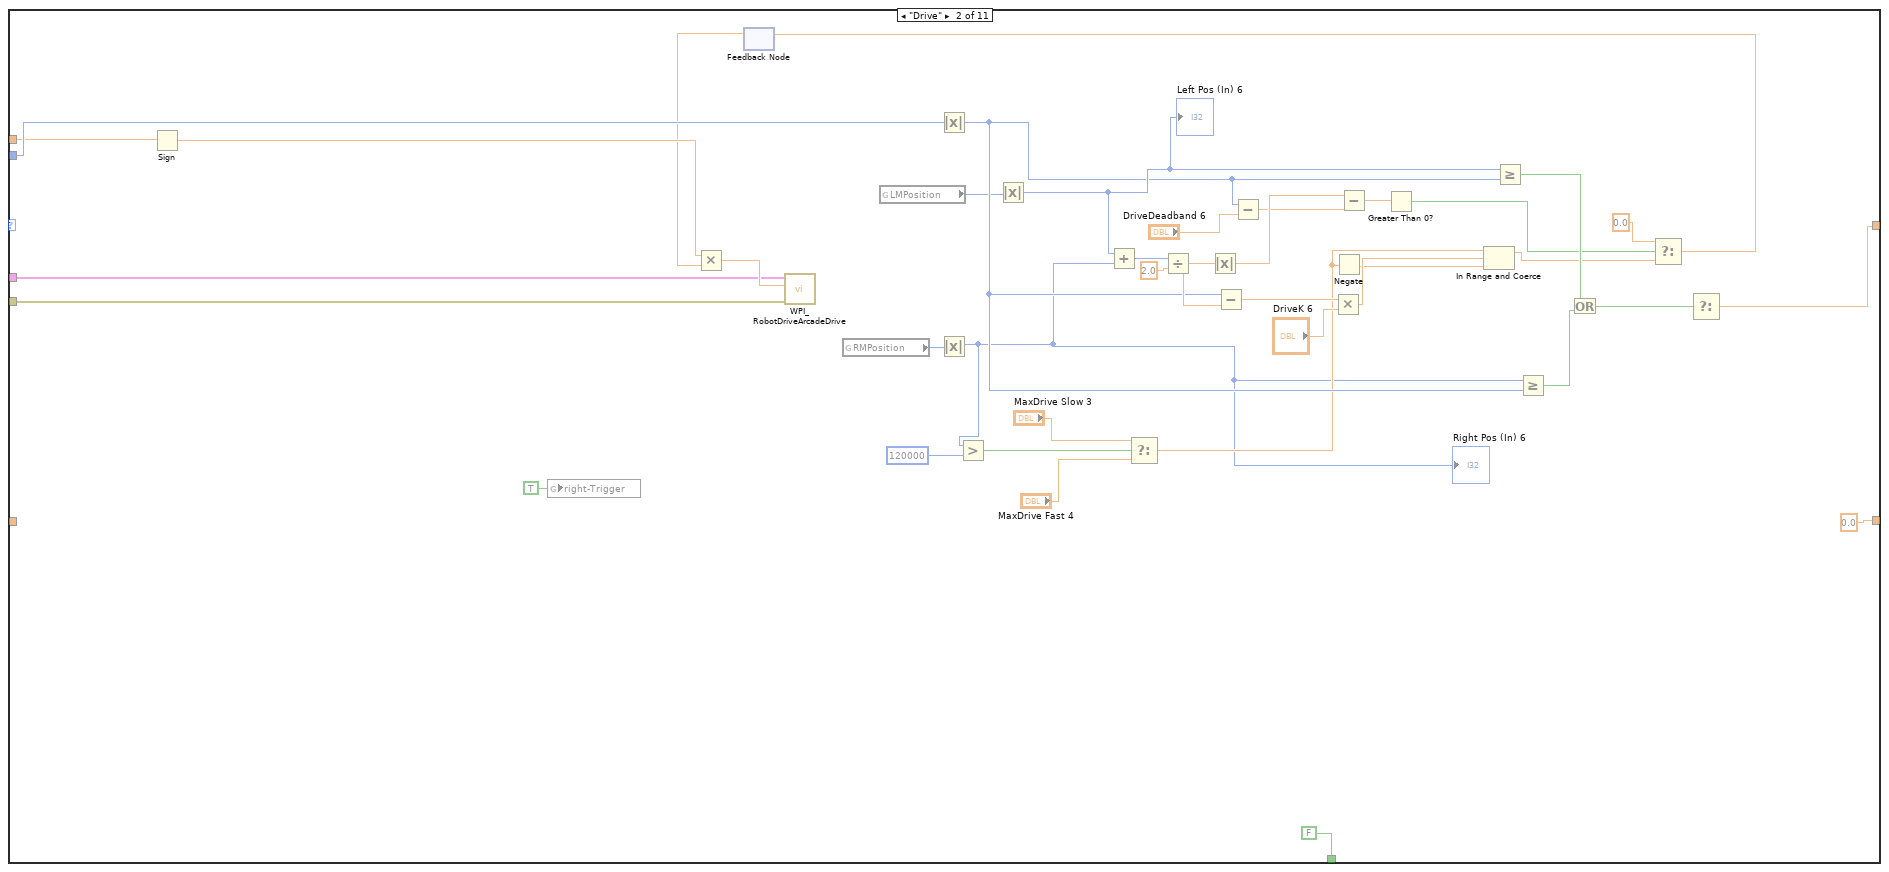
[diagram p19: hidden frame]
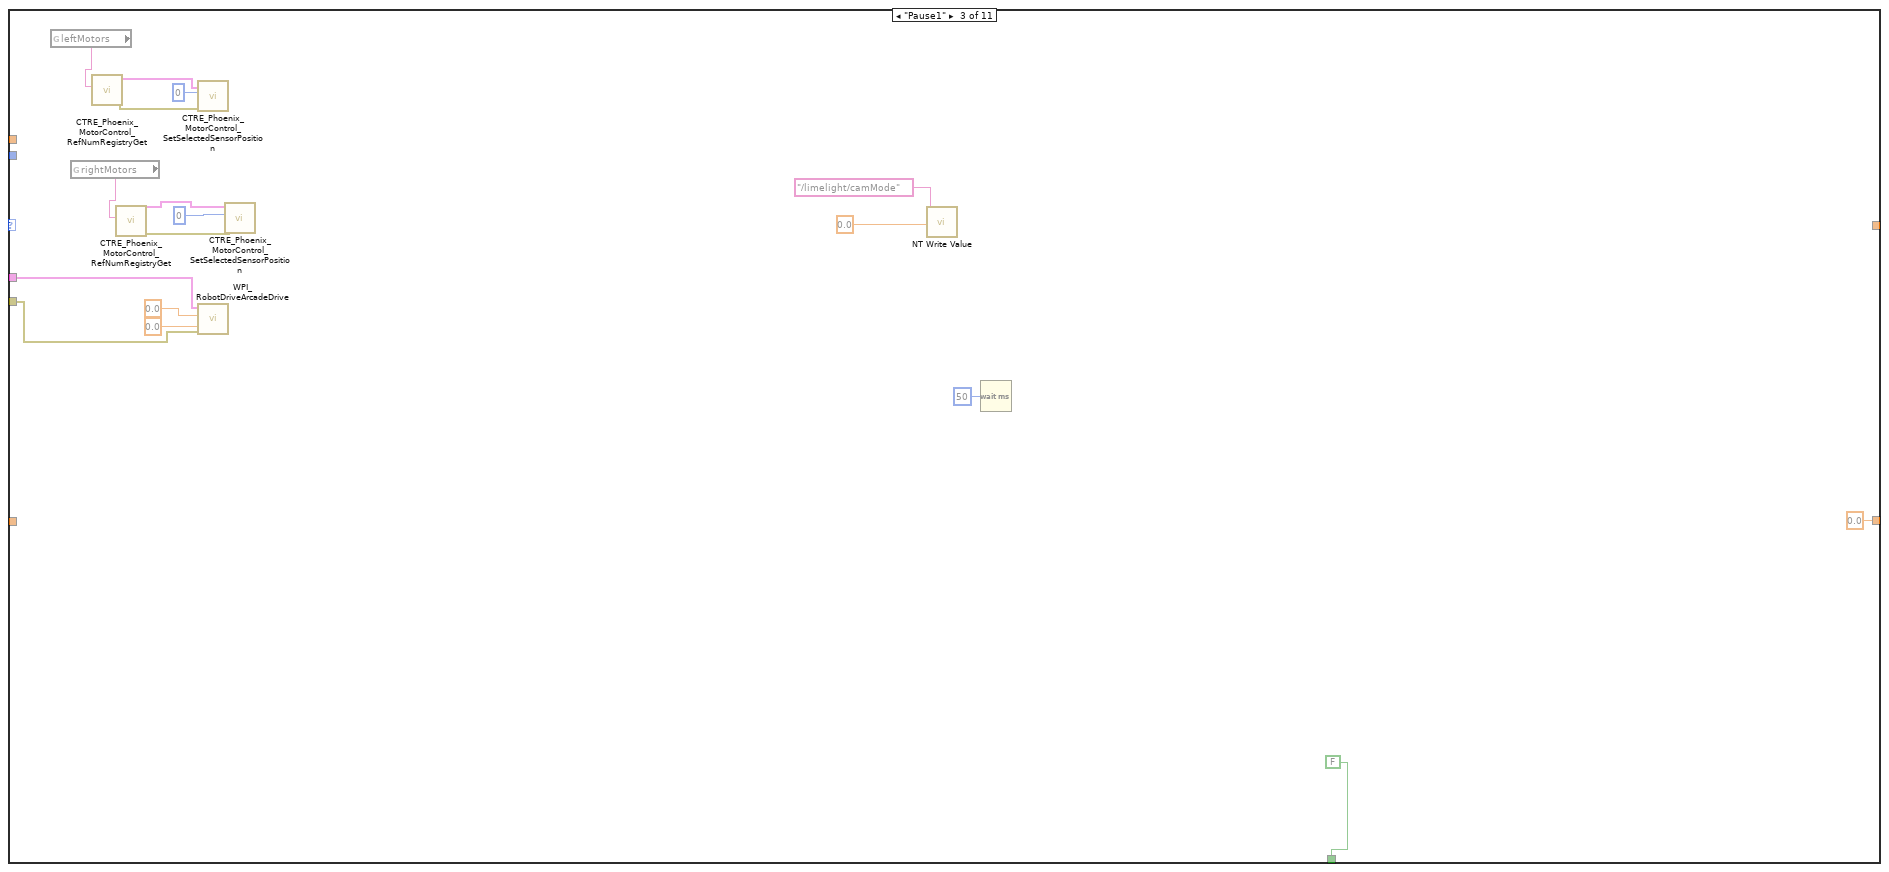
[diagram p20: hidden frame]
diagram:
  (unwired) "This function is run in parallel when the autonomous period begins. It will be terminated automatically when the period ends.\n\nNote that all Driver Station inputs are automatically latched and will not change once auto begins."
  # "The game specific data sent by FMS"
  # "This tells you the autonomous selected in the \ndashboard. Begin.vi publishes the Auto List values\nby writing a constant to the dashboard.\nUpdate the constant to add or modify the name\nof an autonomous."
  # "Every 20ms, report that we are running autonomous\ncode. Loop will abort the same time as the VI."
  # "This gives you the joystick value\nthat is often the throttle"
  # "Use time and/or sensors to control how the robot drives."
  # "This tells you the driver position\nand alliance color"
  n1 = global read "GlobalRefnum.vi" "leftStick"() -> (w1:string)
  n2 = call <vilib>:"WPI_DriverStationGame Specific Data.vi"() -> ("Game Specific Data"=w2:string)  [unwired: 11 in]
  n3 = call <vilib>:"WPI_DriverStationGet Alliance Info.vi"() -> ()  [unwired: 12 out]
  n4 = while {
    stop <- FALSE stop-if-true
    n5 = call <vilib>:"WPI_DriverStationReport Robot Code State.vi"("Autonomous"=TRUE) -> ()  [unwired: 10 in, 1 out]
    n6 = Wait (ms)(milliseconds to wait=u32 20) -> ()  [unwired: 1 out]
  }
  n7 = call <vilib>:"WPI_JoystickRefNum Registry Get.vi"("refnum name"=w1) -> ("JoystickDevRef"=w8:T4)  [unwired: 1 in, 9 out]
  n8 = call <vilib>:"WPI_JoystickGetValues.vi"("JoystickDevRef"=w8) -> ("Axes"=w4:dbl[])  [unwired: 6 in, 4 out]
  n9 = call-poly <vilib>:"NT Read Value.vi"("Name"="Auto Selector") -> ("String"=w5:string)  [unwired: 9 in, 1 out]
  n10 = call-poly <vilib>:"NT Write Value.vi"("Numeric Array"=w4, "Name"="leftStick/Axes") -> ()  [unwired: 9 in, 1 out]
  n11 = Index Array(array=w4, index=2) -> ()  [unwired: 1 out]
  n12 = case shown="\"ShootAndDrive\"" w5 {
    tunnel: w2 -> [_ _ _ _ _ _ _ _ _]
    frame Default {
      n13 = global read "GlobalRefnum.vi" "leftMotors"() -> (w33:string)
      n14 = global read "GlobalRefnum.vi" "rightMotors"() -> (w32:string)
      n15 = Negate(x="Output") -> (-x=w12:dbl)
      n16 = call <vilib>:"CTRE_Phoenix_MotorControl_RefNumRegistryGet.vi"("refnum name"=w33) -> ("error out"=w19:errorcluster, "PhoenixMotorControlDevRef"=w29:T9)  [unwired: 9 in]
      n17 = call <vilib>:"CTRE_Phoenix_MotorControl_RefNumRegistryGet.vi"("refnum name"=w32) -> ("error out"=w20:errorcluster, "PhoenixMotorControlDevRef"=w28:T9)  [unwired: 9 in]
      n18 = Multiply(x="Travel Distance (In)", y=217.29) -> (x*y=w14:dbl)
      n19 = call <vilib>:"CTRE_Phoenix_MotorControl_SetSelectedSensorPosition.vi"("error in (no error)"=w19, "New Sensor Position"=0, "PhoenixMotorControlDevRef"=w29) -> ("error out"=w22:errorcluster, "PhoenixMotorControlDevRef"=w24:T9)  [unwired: 7 in]
      n20 = Select(t=w12, s="Reverse?", f="Output") -> (s? t:f=w15:dbl)
      n21 = Wait (ms)(milliseconds to wait=u32 100) -> ()  [unwired: 1 out]
      n22 = call <vilib>:"CTRE_Phoenix_MotorControl_SetSelectedSensorPosition.vi"("error in (no error)"=w20, "New Sensor Position"=0, "PhoenixMotorControlDevRef"=w28) -> ("error out"=w21:errorcluster, "PhoenixMotorControlDevRef"=w23:T9)  [unwired: 7 in]
      n23 = while {
        tunnel: w24 -> [w42]
        tunnel: w23 -> [w41]
        tunnel: w22 -> [w40]
        tunnel: w21 -> [w39]
        shift-right: [w38] -> _
        shift-left: enum16{"Drive", "End", "Init"}."Init" -> [w44]
        shift-right: [w36] -> _
        shift-left: 0.0 ("y") -> [w37]
        tunnel: w15 -> [w35]
        tunnel: w14 -> [w34]
        stop <- w43 stop-if-true
        n24 = case shown="\"Init\", Default" w44 {
          tunnel: [FALSE FALSE TRUE] -> w43
          tunnel: w42 -> [w60 w90 _]
          tunnel: w41 -> [w57 w89 _]
          tunnel: w40 -> [w59 w88 _]
          tunnel: w39 -> [w56 w87 _]
          tunnel: [w50 w69 enum16{"Drive", "End", "Init"}."End"] -> w38
          tunnel: w37 -> [w53 _ _]
          tunnel: [w49 0.0 0.0] -> w36
          tunnel: w35 -> [_ w64 _]
          tunnel: w34 -> [_ w63 _]
          frame "Init", Default {
            n25 = call <vilib>:"CTRE_Phoenix_MotorControl_SetSelectedSensorPosition.vi"("error in (no error)"=w59, "New Sensor Position"=0, "PhoenixMotorControlDevRef"=w60) -> ()  [unwired: 7 in, 2 out]
            n26 = call <vilib>:"CTRE_Phoenix_MotorControl_SetSelectedSensorPosition.vi"("error in (no error)"=w56, "New Sensor Position"=0, "PhoenixMotorControlDevRef"=w57) -> ()  [unwired: 7 in, 2 out]
            n27 = Add(x=1.0, y=w53) -> (x+y=w49:dbl)
            n28 = Greater Or Equal?(x=w49, y=10.0) -> (x >= y?=w48:bool)
            n29 = global write "Global Vars.vi" "Movement Selector"(enum16{"Teleop", "Nothin"}."Nothin" ("Movement Selector")) -> ()
            n30 = Select(t=enum16{"Drive", "End", "Init"}."Drive", s=w48, f=enum16{"Drive", "End", "Init"}."Init") -> (s? t:f=w50:enum16{"Drive", "End", "Init"})
          }
          frame "Drive" {
            w86 = T14 0 items=["PercentOutput"=0, "Position"=1, "Velocity"=2, "Current"=3, "Follower"=5, "MotionProfile"=6, "MotionMagic"=7, "MotionProfileArc"=10, "Disabled"=15] ("Control Mode")
            n31 = Negate(x=w64) -> (-x=w85:dbl)
            n32 = call <vilib>:"CTRE_Phoenix_MotorControl_Set.vi"("error in (no error)"=w88, "Output"=w64, "Control Mode"=w86, "PhoenixMotorControlDevRef"=w90) -> ("error out"=w82:errorcluster, "PhoenixMotorControlDevRef"=w81:T9)  [unwired: 6 in]
            n33 = call <vilib>:"CTRE_Phoenix_MotorControl_Set.vi"("error in (no error)"=w87, "Output"=w85, "Control Mode"=w86, "PhoenixMotorControlDevRef"=w89) -> ("error out"=w83:errorcluster, "PhoenixMotorControlDevRef"=w84:T9)  [unwired: 6 in]
            n34 = call-poly <vilib>:"CTRE_Phoenix_MotorController_Get_TalonFX.vi"("PhoenixMotorControlDevRef"=w84, "error in"=w83) -> ("Position (Raw Sensor Units)"=w79:i32)  [unwired: 10 in, 3 out]
            n35 = call-poly <vilib>:"CTRE_Phoenix_MotorController_Get_TalonFX.vi"("PhoenixMotorControlDevRef"=w81, "error in"=w82) -> ("Position (Raw Sensor Units)"=w80:i32)  [unwired: 10 in, 3 out]
            n36 = Absolute Value(x=w63) -> (abs(x)=w65:dbl)
            n37 = global write "Global Vars.vi" "Movement Selector"(enum16{"Teleop", "Nothin"}."Nothin" ("Movement Selector")) -> ()
            n38 = Absolute Value(x=w79) -> (abs(x)=w77:i32)
            n39 = Absolute Value(x=w80) -> (abs(x)=w74:i32)
            n40 = Greater Or Equal?(x=w74, y=w65) -> (x >= y?=w72:bool)
            n41 = Greater Or Equal?(x=w77, y=w65) -> (x >= y?=w71:bool)
            n42 = Divide(x=w77, y=217.29) -> (x/y=→"Right Pos (In)":dbl)
            n43 = Divide(x=w74, y=217.29) -> (x/y=→"Left Pos (In)":dbl)
            n44 = Or(x=w72, y=w71) -> (x .or. y?=w70:bool)
            n45 = Select(t=enum16{"Drive", "End", "Init"}."End", s=w70, f=enum16{"Drive", "End", "Init"}."Drive") -> (s? t:f=w69:enum16{"Drive", "End", "Init"})
          }
          frame "End" {
            n46 = global write "Global Vars.vi" "Movement Selector"(enum16{"Teleop", "Nothin"}."Teleop" ("Movement Selector")) -> ()
          }
        }
        n47 = Wait (ms)(milliseconds to wait=u32 10) -> ()  [unwired: 1 out]
      }
    }
    frame "DriveKp" {
      w98 = 1.0
      n48 = global read "GlobalRefnum.vi" "leftMotors"() -> (w117:string)
      n49 = global read "GlobalRefnum.vi" "rightMotors"() -> (w116:string)
      n50 = Negate(x=w98) -> (-x=w99:dbl)
      n51 = call <vilib>:"CTRE_Phoenix_MotorControl_RefNumRegistryGet.vi"("refnum name"=w117) -> ("error out"=w104:errorcluster, "PhoenixMotorControlDevRef"=w114:T9)  [unwired: 9 in]
      n52 = global read "GlobalRefnum.vi" "twoMotorDrive"() -> (w97:string)
      n53 = call <vilib>:"CTRE_Phoenix_MotorControl_RefNumRegistryGet.vi"("refnum name"=w116) -> ("error out"=w105:errorcluster, "PhoenixMotorControlDevRef"=w113:T9)  [unwired: 9 in]
      n54 = call <vilib>:"CTRE_Phoenix_MotorControl_SetSelectedSensorPosition.vi"("error in (no error)"=w104, "New Sensor Position"=0, "PhoenixMotorControlDevRef"=w114) -> ("error out"=w107:errorcluster, "PhoenixMotorControlDevRef"=w109:T9)  [unwired: 7 in]
      n55 = Select(t=w99, s="Reverse? 2", f=w98) -> (s? t:f=w100:dbl)
      n56 = Wait (ms)(milliseconds to wait=u32 100) -> ()  [unwired: 1 out]
      n57 = call <vilib>:"WPI_RobotDriveRefNum Registry Get.vi"("refnum name"=w97) -> ("RobotDriveDevRef"=w96:T15)  [unwired: 9 in, 1 out]
      n58 = call <vilib>:"CTRE_Phoenix_MotorControl_SetSelectedSensorPosition.vi"("error in (no error)"=w105, "New Sensor Position"=0, "PhoenixMotorControlDevRef"=w113) -> ("error out"=w106:errorcluster, "PhoenixMotorControlDevRef"=w108:T9)  [unwired: 7 in]
      n59 = while {
        tunnel: w109 -> [w127]
        tunnel: w108 -> [w126]
        tunnel: w107 -> [w125]
        tunnel: w106 -> [w124]
        shift-right: [w123] -> _
        shift-left: enum16{"Drive", "End", "Init"}."Init" -> [w129]
        shift-right: [w121] -> _
        shift-left: 0.0 ("y") -> [w122]
        tunnel: w100 -> [w120]
        tunnel: "Travel Distance (In) 2" -> [w119]
        tunnel: w96 -> [w118]
        stop <- w128 stop-if-true
        n60 = case shown="\"Drive\"" w129 {
          tunnel: [FALSE FALSE TRUE] -> w128
          tunnel: w127 -> [w145 w185 _]
          tunnel: w126 -> [w142 w184 _]
          tunnel: w125 -> [w144 w183 _]
          tunnel: w124 -> [w141 w182 _]
          tunnel: [w135 w176 enum16{"Drive", "End", "Init"}."End"] -> w123
          tunnel: w122 -> [w138 _ _]
          tunnel: [w134 0.0 0.0] -> w121
          tunnel: w120 -> [_ w160 _]
          tunnel: w119 -> [_ w172 _]
          tunnel: w118 -> [_ w148 _]
          frame "Init", Default {
            n61 = global write "Global Vars.vi" "Movement Selector"(enum16{"Teleop", "Nothin"}."Nothin" ("Movement Selector")) -> ()
            n62 = call <vilib>:"CTRE_Phoenix_MotorControl_SetSelectedSensorPosition.vi"("error in (no error)"=w144, "New Sensor Position"=0, "PhoenixMotorControlDevRef"=w145) -> ()  [unwired: 7 in, 2 out]
            n63 = call <vilib>:"CTRE_Phoenix_MotorControl_SetSelectedSensorPosition.vi"("error in (no error)"=w141, "New Sensor Position"=0, "PhoenixMotorControlDevRef"=w142) -> ()  [unwired: 7 in, 2 out]
            n64 = Add(x=1.0, y=w138) -> (x+y=w134:dbl)
            n65 = Greater Or Equal?(x=w134, y=10.0) -> (x >= y?=w133:bool)
            n66 = Select(t=enum16{"Drive", "End", "Init"}."Drive", s=w133, f=enum16{"Drive", "End", "Init"}."Init") -> (s? t:f=w135:enum16{"Drive", "End", "Init"})
          }
          frame "Drive" {
            n67 = global write "Global Vars.vi" "Movement Selector"(enum16{"Teleop", "Nothin"}."Nothin" ("Movement Selector")) -> ()
            n68 = Sign(1:w160) -> (0:w159:dbl)
            n69 = feedback #1() -> (w153:dbl)  [unwired: 1 in]
            n70 = Multiply(x=w159, y=w153) -> (x*y=w147:dbl)
            n71 = call-poly <vilib>:"WPI_RobotDriveArcadeDrive.vi"("X axis value"=w147, "RobotDriveDevRef"=w148) -> ()  [unwired: 7 in, 3 out]
            n72 = call-poly <vilib>:"CTRE_Phoenix_MotorController_Get_TalonFX.vi"("PhoenixMotorControlDevRef"=w184, "error in"=w182) -> ("Position (Raw Sensor Units)"=w180:i32)  [unwired: 10 in, 3 out]
            n73 = call-poly <vilib>:"CTRE_Phoenix_MotorController_Get_TalonFX.vi"("PhoenixMotorControlDevRef"=w185, "error in"=w183) -> ("Position (Raw Sensor Units)"=w181:i32)  [unwired: 10 in, 3 out]
            n74 = Absolute Value(x=w172) -> (abs(x)=w151:i32)
            n75 = Absolute Value(x=w180) -> (abs(x)=w152:i32)
            "Right Pos (In) 2" <- w152
            n76 = Absolute Value(x=w181) -> (abs(x)=w163:i32)
            "Left Pos (In) 2" <- w163
            n77 = Add(x=w163, y=w152) -> (x+y=w165:i32)
            n78 = Divide(x=w165, y=2.0) -> (x/y=w162:dbl)
            n79 = Absolute Value(x=w162) -> (abs(x)=w167:dbl)
            n80 = Subtract(x=w151, y=w162) -> (x-y=w171:dbl)
            n81 = Subtract(x=w151, y="DriveDeadband") -> (x-y=w157:dbl)
            n82 = Negate(x="MaxDrive") -> (-x=w168:dbl)
            n83 = Multiply(x=w171, y="DriveK") -> (x*y=w170:dbl)
            n84 = Subtract(x=w167, y=w157) -> (x-y=w156:dbl)
            n85 = Greater Than 0?(x=w156) -> (x > 0?=w155:bool)
            n86 = In Range and Coerce(upper limit="MaxDrive", x=w170, lower limit=w168) -> (coerced(x)=w150:dbl)  [unwired: 1 out]
            n87 = Greater Or Equal?(x=w163, y=w151) -> (x >= y?=w179:bool)
            n88 = Greater Or Equal?(x=w152, y=w151) -> (x >= y?=w178:bool)
            n89 = Or(x=w179, y=w178) -> (x .or. y?=w177:bool)
            n90 = Select(t=0.0, s=w155, f=w150) -> (s? t:f=w154:dbl)
            n91 = feedback-in #1(w154) -> ()
            n92 = Select(t=enum16{"Drive", "End", "Init"}."End", s=w177, f=enum16{"Drive", "End", "Init"}."Drive") -> (s? t:f=w176:enum16{"Drive", "End", "Init"})
          }
          frame "End" {
            n93 = global write "Global Vars.vi" "Movement Selector"(enum16{"Teleop", "Nothin"}."Teleop" ("Movement Selector")) -> ()
          }
        }
        n94 = Wait (ms)(milliseconds to wait=u32 10) -> ()  [unwired: 1 out]
      }
    }
    frame "ShootAndDrive" {
      w191 = 1.0
      n95 = global read "GlobalRefnum.vi" "leftMotors"() -> (w210:string)
      n96 = global read "GlobalRefnum.vi" "rightMotors"() -> (w209:string)
      n97 = Negate(x=w191) -> (-x=w192:dbl)
      n98 = call <vilib>:"CTRE_Phoenix_MotorControl_RefNumRegistryGet.vi"("refnum name"=w210) -> ("error out"=w197:errorcluster, "PhoenixMotorControlDevRef"=w207:T9)  [unwired: 9 in]
      n99 = call <vilib>:"CTRE_Phoenix_MotorControl_RefNumRegistryGet.vi"("refnum name"=w209) -> ("error out"=w198:errorcluster, "PhoenixMotorControlDevRef"=w206:T9)  [unwired: 9 in]
      n100 = call <vilib>:"CTRE_Phoenix_MotorControl_SetSelectedSensorPosition.vi"("error in (no error)"=w197, "New Sensor Position"=0, "PhoenixMotorControlDevRef"=w207) -> ("error out"=w200:errorcluster, "PhoenixMotorControlDevRef"=w202:T9)  [unwired: 7 in]
      n101 = Select(t=w192, s="Reverse? 3", f=w191) -> (s? t:f=w193:dbl)
      n102 = Wait (ms)(milliseconds to wait=u32 100) -> ()  [unwired: 1 out]
      n103 = call <vilib>:"CTRE_Phoenix_MotorControl_SetSelectedSensorPosition.vi"("error in (no error)"=w198, "New Sensor Position"=0, "PhoenixMotorControlDevRef"=w206) -> ("error out"=w199:errorcluster, "PhoenixMotorControlDevRef"=w201:T9)  [unwired: 7 in]
      n104 = while {
        tunnel: w202 -> [w219]
        tunnel: w201 -> [w218]
        tunnel: w200 -> [w217]
        tunnel: w199 -> [w216]
        shift-right: [w215] -> _
        shift-left: enum16{"Drive", "End", "Init", "Shoot"}."Init" -> [w221]
        shift-right: [w213] -> _
        shift-left: 0.0 ("y") -> [w214]
        tunnel: w193 -> [w212]
        tunnel: "Travel Distance (In) 3" -> [w211]
        stop <- w220 stop-if-true
        n105 = case shown="\"Init\", Default" w221 {
          tunnel: [FALSE FALSE FALSE TRUE] -> w220
          tunnel: w219 -> [w238 w282 _ w291]
          tunnel: w218 -> [w235 w281 _ w296]
          tunnel: w217 -> [w237 w280 _ w290]
          tunnel: w216 -> [w234 w279 _ w294]
          tunnel: [w229 w268 enum16{"Drive", "End", "Init", "Shoot"}."End" enum16{"Drive", "End", "Init", "Shoot"}."End"] -> w215
          tunnel: w214 -> [w231 _ _ _]
          tunnel: [w228 0.0 0.0 0.0] -> w213
          tunnel: w212 -> [_ w254 _ _]
          tunnel: w211 -> [_ w266 _ _]
          frame "Init", Default {
            n106 = call <vilib>:"CTRE_Phoenix_MotorControl_SetSelectedSensorPosition.vi"("error in (no error)"=w237, "New Sensor Position"=0, "PhoenixMotorControlDevRef"=w238) -> ()  [unwired: 7 in, 2 out]
            n107 = call <vilib>:"CTRE_Phoenix_MotorControl_SetSelectedSensorPosition.vi"("error in (no error)"=w234, "New Sensor Position"=0, "PhoenixMotorControlDevRef"=w235) -> ()  [unwired: 7 in, 2 out]
            n108 = global write "Global Vars.vi" "Manual Shooter Speed"(14500.0 ("Manual Shooter Speed")) -> ()
            n109 = global write "Joystick_Buttons.vi" "left-ThumbR"(TRUE ("left-ThumbR")) -> ()
            n110 = Add(x=1.0, y=w231) -> (x+y=w228:dbl)
            n111 = Greater Or Equal?(x=w228, y=200.0) -> (x >= y?=w227:bool)
            n112 = Select(t=enum16{"Drive", "End", "Init", "Shoot"}."Drive", s=w227, f=enum16{"Drive", "End", "Init", "Shoot"}."Init") -> (s? t:f=w229:enum16{"Drive", "End", "Init", "Shoot"})
          }
          frame "Drive" {
            w278 = T14 0 items=["PercentOutput"=0, "Position"=1, "Velocity"=2, "Current"=3, "Follower"=5, "MotionProfile"=6, "MotionMagic"=7, "MotionProfileArc"=10, "Disabled"=15] ("Control Mode")
            n113 = Sign(1:w254) -> (0:w253:dbl)
            n114 = feedback #2() -> (w245:dbl)  [unwired: 1 in]
            n115 = Multiply(x=w253, y=w245) -> (x*y=w252:dbl)
            n116 = Negate(x=w252) -> (-x=w277:dbl)
            n117 = call <vilib>:"CTRE_Phoenix_MotorControl_Set.vi"("error in (no error)"=w279, "Output"=w277, "Control Mode"=w278, "PhoenixMotorControlDevRef"=w281) -> ("error out"=w276:errorcluster, "PhoenixMotorControlDevRef"=w247:T9)  [unwired: 6 in]
            n118 = call <vilib>:"CTRE_Phoenix_MotorControl_Set.vi"("error in (no error)"=w280, "Output"=w252, "Control Mode"=w278, "PhoenixMotorControlDevRef"=w282) -> ("error out"=w275:errorcluster, "PhoenixMotorControlDevRef"=w274:T9)  [unwired: 6 in]
            n119 = call-poly <vilib>:"CTRE_Phoenix_MotorController_Get_TalonFX.vi"("PhoenixMotorControlDevRef"=w247, "error in"=w276) -> ("Position (Raw Sensor Units)"=w272:i32)  [unwired: 10 in, 3 out]
            n120 = call-poly <vilib>:"CTRE_Phoenix_MotorController_Get_TalonFX.vi"("PhoenixMotorControlDevRef"=w274, "error in"=w275) -> ("Position (Raw Sensor Units)"=w273:i32)  [unwired: 10 in, 3 out]
            n121 = Absolute Value(x=w266) -> (abs(x)=w244:i32)
            n122 = Absolute Value(x=w272) -> (abs(x)=w242:i32)
            "Right Pos (In) 3" <- w242
            n123 = Absolute Value(x=w273) -> (abs(x)=w257:i32)
            "Left Pos (In) 3" <- w257
            n124 = Add(x=w257, y=w242) -> (x+y=w259:i32)
            n125 = Divide(x=w259, y=2.0) -> (x/y=w256:dbl)
            n126 = Absolute Value(x=w256) -> (abs(x)=w261:dbl)
            n127 = Subtract(x=w244, y=w256) -> (x-y=w265:dbl)
            n128 = Subtract(x=w244, y="DriveDeadband 2") -> (x-y=w250:dbl)
            n129 = Negate(x="MaxDrive 2") -> (-x=w262:dbl)
            n130 = Multiply(x=w265, y="DriveK 2") -> (x*y=w264:dbl)
            n131 = Subtract(x=w261, y=w250) -> (x-y=w249:dbl)
            n132 = Greater Than 0?(x=w249) -> (x > 0?=w248:bool)
            n133 = In Range and Coerce(upper limit="MaxDrive 2", x=w264, lower limit=w262) -> (coerced(x)=w243:dbl)  [unwired: 1 out]
            n134 = Greater Or Equal?(x=w257, y=w244) -> (x >= y?=w271:bool)
            n135 = Greater Or Equal?(x=w242, y=w244) -> (x >= y?=w270:bool)
            n136 = Or(x=w271, y=w270) -> (x .or. y?=w269:bool)
            n137 = Select(t=0.0, s=w248, f=w243) -> (s? t:f=w246:dbl)
            n138 = feedback-in #2(w246) -> ()
            n139 = Select(t=enum16{"Drive", "End", "Init", "Shoot"}."Shoot", s=w269, f=enum16{"Drive", "End", "Init", "Shoot"}."Drive") -> (s? t:f=w268:enum16{"Drive", "End", "Init", "Shoot"})
          }
          frame "Shoot" {
            n140 = global write "Joystick_Buttons.vi" "left-Trigger"(TRUE ("left-ThumbR")) -> ()
            n141 = Wait (ms)(milliseconds to wait=u32 3000) -> ()  [unwired: 1 out]
          }
          frame "End" {
            w292 = T14 0 items=["PercentOutput"=0, "Position"=1, "Velocity"=2, "Current"=3, "Follower"=5, "MotionProfile"=6, "MotionMagic"=7, "MotionProfileArc"=10, "Disabled"=15] ("Control Mode")
            w295 = T14 0 items=["PercentOutput"=0, "Position"=1, "Velocity"=2, "Current"=3, "Follower"=5, "MotionProfile"=6, "MotionMagic"=7, "MotionProfileArc"=10, "Disabled"=15] ("Control Mode")
            n142 = call <vilib>:"CTRE_Phoenix_MotorControl_Set.vi"("error in (no error)"=w290, "Output"=0.0, "Control Mode"=w292, "PhoenixMotorControlDevRef"=w291) -> ()  [unwired: 6 in, 2 out]
            n143 = call <vilib>:"CTRE_Phoenix_MotorControl_Set.vi"("error in (no error)"=w294, "Output"=0.0, "Control Mode"=w295, "PhoenixMotorControlDevRef"=w296) -> ()  [unwired: 6 in, 2 out]
          }
        }
        n144 = Wait (ms)(milliseconds to wait=u32 10) -> ()  [unwired: 1 out]
      }
    }
    frame "5BallOurTrench" {
      w304 = 1.0
      n145 = Negate(x=w304) -> (-x=w305:dbl)
      n146 = global read "GlobalRefnum.vi" "twoMotorDrive"() -> (w303:string)
      n147 = Select(t=w305, s="Reverse? 4", f=w304) -> (s? t:f=w306:dbl)
      n148 = Wait (ms)(milliseconds to wait=u32 100) -> ()  [unwired: 1 out]
      n149 = call <vilib>:"WPI_RobotDriveRefNum Registry Get.vi"("refnum name"=w303) -> ("error out"=w301:errorcluster, "RobotDriveDevRef"=w302:T15)  [unwired: 9 in]
      n150 = while {
        shift-right: [w311] -> _
        shift-left: T6."Init" -> [w312]
        shift-right: [w317] -> _
        shift-left: 0.0 ("y") -> [w318]
        tunnel: w306 -> [w316]
        tunnel: "Travel Distance (In) 4" -> [w315]
        tunnel: w302 -> [w314]
        tunnel: w301 -> [w313]
        stop <- w319 stop-if-true
        n151 = case shown="\"Init\", Default" w312 {
          tunnel: [FALSE FALSE FALSE FALSE FALSE TRUE] -> w319
          tunnel: w318 -> [w337 _ _ w401 _ _]
          tunnel: [w336 0.0 0.0 w402 0.0 0.0] -> w317
          tunnel: w316 -> [_ w364 _ _ _ _]
          tunnel: w315 -> [_ w375 _ _ _ _]
          tunnel: w314 -> [_ w353 w387 w413 w422 w445]
          tunnel: w313 -> [_ w352 w386 w412 w421 w444]
          tunnel: [w323 w347 T6."Aim" w408 T6."End" T6."End"] -> w311
          frame "Init", Default {
            n152 = global read "GlobalRefnum.vi" "leftMotors"() -> (w329:string)
            n153 = global read "GlobalRefnum.vi" "rightMotors"() -> (w328:string)
            n154 = call <vilib>:"CTRE_Phoenix_MotorControl_RefNumRegistryGet.vi"("refnum name"=w329) -> ("error out"=w330:errorcluster, "PhoenixMotorControlDevRef"=w331:T9)  [unwired: 9 in]
            n155 = call <vilib>:"CTRE_Phoenix_MotorControl_RefNumRegistryGet.vi"("refnum name"=w328) -> ("error out"=w326:errorcluster, "PhoenixMotorControlDevRef"=w327:T9)  [unwired: 9 in]
            n156 = call <vilib>:"CTRE_Phoenix_MotorControl_SetSelectedSensorPosition.vi"("error in (no error)"=w330, "New Sensor Position"=0, "PhoenixMotorControlDevRef"=w331) -> ()  [unwired: 7 in, 2 out]
            n157 = call <vilib>:"CTRE_Phoenix_MotorControl_SetSelectedSensorPosition.vi"("error in (no error)"=w326, "New Sensor Position"=0, "PhoenixMotorControlDevRef"=w327) -> ()  [unwired: 7 in, 2 out]
            n158 = call-poly <vilib>:"NT Write Value.vi"("Numeric"=3.0, "Name"="/limelight/ledMode") -> ()  [unwired: 9 in, 1 out]
            n159 = Add(x=1.0, y=w337) -> (x+y=w336:dbl)
            n160 = Greater Or Equal?(x=w336, y=10.0) -> (x >= y?=w335:bool)
            n161 = Select(t=T6."Drive", s=w335, f=T6."Init") -> (s? t:f=w323:T6)
          }
          frame "Drive" {
            n162 = Sign(1:w364) -> (0:w363:dbl)
            n163 = global write "Joystick_Buttons.vi" "right-Trigger"(TRUE ("left-ThumbR")) -> ()
            n164 = feedback #3() -> (w357:dbl)  [unwired: 1 in]
            n165 = Multiply(x=w363, y=w357) -> (x*y=w354:dbl)
            n166 = call-poly <vilib>:"WPI_RobotDriveArcadeDrive.vi"("error in (no error)"=w352, "X axis value"=w354, "RobotDriveDevRef"=w353) -> ()  [unwired: 6 in, 3 out]
            n167 = global read "Global Vars.vi" "RMPosition"() -> (w343:i32)
            n168 = global read "Global Vars.vi" "LMPosition"() -> (w351:i32)
            n169 = Absolute Value(x=w375) -> (abs(x)=w356:i32)
            n170 = Absolute Value(x=w343) -> (abs(x)=w340:i32)
            "Right Pos (In) 4" <- w340
            n171 = Greater?(x=w340, y=120000) -> (0:w341:bool)
            n172 = Absolute Value(x=w351) -> (abs(x)=w367:i32)
            "Left Pos (In) 4" <- w367
            n173 = Add(x=w367, y=w340) -> (x+y=w369:i32)
            n174 = Select(t="MaxDrive Slow", s=w341, f="MaxDrive Fast") -> (s? t:f=w344:dbl)
            n175 = Divide(x=w369, y=2.0) -> (x/y=w366:dbl)
            n176 = Absolute Value(x=w366) -> (abs(x)=w371:dbl)
            n177 = Subtract(x=w356, y=w366) -> (x-y=w374:dbl)
            n178 = Subtract(x=w356, y="DriveDeadband 3") -> (x-y=w361:dbl)
            n179 = Multiply(x=w374, y="DriveK 3") -> (x*y=w373:dbl)
            n180 = Negate(x=w344) -> (-x=w372:dbl)
            n181 = Subtract(x=w371, y=w361) -> (x-y=w360:dbl)
            n182 = Greater Than 0?(x=w360) -> (x > 0?=w359:bool)
            n183 = In Range and Coerce(upper limit=w344, x=w373, lower limit=w372) -> (coerced(x)=w355:dbl)  [unwired: 1 out]
            n184 = Greater Or Equal?(x=w367, y=w356) -> (x >= y?=w379:bool)
            n185 = Greater Or Equal?(x=w340, y=w356) -> (x >= y?=w378:bool)
            n186 = Or(x=w379, y=w378) -> (x .or. y?=w377:bool)
            n187 = Select(t=0.0, s=w359, f=w355) -> (s? t:f=w358:dbl)
            n188 = feedback-in #3(w358) -> ()
            n189 = Select(t=T6."Pause1", s=w377, f=T6."Drive") -> (s? t:f=w347:T6)
          }
          frame "Pause1" {
            n190 = global read "GlobalRefnum.vi" "leftMotors"() -> (w393:string)
            n191 = global read "GlobalRefnum.vi" "rightMotors"() -> (w392:string)
            n192 = call <vilib>:"CTRE_Phoenix_MotorControl_RefNumRegistryGet.vi"("refnum name"=w393) -> ("error out"=w394:errorcluster, "PhoenixMotorControlDevRef"=w395:T9)  [unwired: 9 in]
            n193 = call <vilib>:"CTRE_Phoenix_MotorControl_RefNumRegistryGet.vi"("refnum name"=w392) -> ("error out"=w390:errorcluster, "PhoenixMotorControlDevRef"=w391:T9)  [unwired: 9 in]
            n194 = call <vilib>:"CTRE_Phoenix_MotorControl_SetSelectedSensorPosition.vi"("error in (no error)"=w394, "New Sensor Position"=0, "PhoenixMotorControlDevRef"=w395) -> ()  [unwired: 7 in, 2 out]
            n195 = call-poly <vilib>:"WPI_RobotDriveArcadeDrive.vi"("error in (no error)"=w386, "Y axis value"=0.0, "X axis value"=0.0, "RobotDriveDevRef"=w387) -> ()  [unwired: 5 in, 3 out]
            n196 = call <vilib>:"CTRE_Phoenix_MotorControl_SetSelectedSensorPosition.vi"("error in (no error)"=w390, "New Sensor Position"=0, "PhoenixMotorControlDevRef"=w391) -> ()  [unwired: 7 in, 2 out]
            n197 = call-poly <vilib>:"NT Write Value.vi"("Numeric"=0.0, "Name"="/limelight/camMode") -> ()  [unwired: 9 in, 1 out]
            n198 = Wait (ms)(milliseconds to wait=u32 50) -> ()  [unwired: 1 out]
          }
          frame "Aim" {
            n199 = global write "Joystick_Buttons.vi" "left-ThumbMain"(TRUE ("left-ThumbMain")) -> ()
            n200 = call "Limelight_Differential.vi"() -> ("DriveCommand"=w416:dbl, "SteerCommand"=w417:dbl)  [unwired: 8 in, 1 out]
            n201 = call-poly <vilib>:"NT Write Value.vi"("Numeric"=0.0, "Name"="/limelight/camMode") -> ()  [unwired: 9 in, 1 out]
            n202 = call-poly <vilib>:"NT Write Value.vi"("Numeric"=w417, "Name"="Aim Angle") -> ()  [unwired: 9 in, 1 out]
            n203 = call <vilib>:"WPI_RobotDriveArcadeDrive_Standard(NoSaturation).vi"("error in (no error)"=w412, "Y axis value"=w417, "X axis value"=w416, "RobotDriveDevRef"=w413) -> ("Motor Values"=w411:dbl[])  [unwired: 7 out]
            n204 = call-poly <vilib>:"NT Write Value.vi"("Numeric Array"=w411, "Name"="RobotDrive Motors") -> ()  [unwired: 9 in, 1 out]
            n205 = Add(x=1.0, y=w401) -> (x+y=w402:dbl)
            n206 = Greater Or Equal?(x=w402, y=100.0) -> (x >= y?=w403:bool)
            n207 = Select(t=T6."Shoot", s=w403, f=T6."Aim") -> (s? t:f=w408:T6)
          }
          frame "Shoot" {
            n208 = call "Limelight_Differential.vi"() -> ("DriveCommand"=w426:dbl, "SteerCommand"=w427:dbl)  [unwired: 8 in, 1 out]
            n209 = call-poly <vilib>:"NT Write Value.vi"("Numeric"=w427, "Name"="Aim Angle") -> ()  [unwired: 9 in, 1 out]
            n210 = call <vilib>:"WPI_RobotDriveArcadeDrive_Standard(NoSaturation).vi"("error in (no error)"=w421, "Y axis value"=w427, "X axis value"=w426, "RobotDriveDevRef"=w422) -> ("Motor Values"=w424:dbl[])  [unwired: 7 out]
            n211 = call-poly <vilib>:"NT Write Value.vi"("Numeric Array"=w424, "Name"="RobotDrive Motors") -> ()  [unwired: 9 in, 1 out]
            n212 = global write "Joystick_Buttons.vi" "left-ThumbMain"(TRUE ("left-ThumbMain")) -> ()
            n213 = global write "Joystick_Buttons.vi" "left-Trigger"(TRUE ("left-ThumbR")) -> ()
            n214 = global write "Joystick_Buttons.vi" "right-Trigger"(TRUE ("left-ThumbMain")) -> ()
            n215 = global write "Joystick_Buttons.vi" "left-ThumbR"(TRUE ("left-ThumbMain")) -> ()
            n216 = Wait (ms)(milliseconds to wait=u32 5000) -> ()  [unwired: 1 out]
          }
          frame "End" {
            n217 = call <vilib>:"WPI_RobotDriveArcadeDrive_Standard(NoSaturation).vi"("error in (no error)"=w444, "Y axis value"=0.0, "X axis value"=0.0, "RobotDriveDevRef"=w445) -> ()  [unwired: 8 out]
            n218 = global write "Joystick_Buttons.vi" "right-Trigger"(FALSE ("left-ThumbR")) -> ()
            n219 = global write "Joystick_Buttons.vi" "left-ThumbMain"(FALSE ("left-ThumbMain")) -> ()
            n220 = global write "Joystick_Buttons.vi" "left-ThumbR"(FALSE ("left-ThumbMain")) -> ()
            n221 = global write "Joystick_Buttons.vi" "left-Trigger"(FALSE ("left-ThumbR")) -> ()
            n222 = call-poly <vilib>:"NT Write Value.vi"("Numeric"=1.0, "Name"="/limelight/camMode") -> ()  [unwired: 9 in, 1 out]
            n223 = Wait (ms)(milliseconds to wait=u32 50) -> ()  [unwired: 1 out]
          }
        }
        n224 = Wait (ms)(milliseconds to wait=u32 10) -> ()  [unwired: 1 out]
      }
    }
    frame "6BallOurTrench" {
      n225 = disable-structure shown="Disabled" {
        frame Disabled {
          w451 = 1.0
          n226 = Negate(x=w451) -> (-x=w452:dbl)
          n227 = global read "GlobalRefnum.vi" "twoMotorDrive"() -> (w450:string)
          n228 = Select(t=w452, s="Reverse? 6", f=w451) -> (s? t:f=w453:dbl)
          n229 = Wait (ms)(milliseconds to wait=u32 100) -> ()  [unwired: 1 out]
          n230 = call <vilib>:"WPI_RobotDriveRefNum Registry Get.vi"("refnum name"=w450) -> ("error out"=w448:errorcluster, "RobotDriveDevRef"=w449:T15)  [unwired: 9 in]
          n231 = while {
            shift-right: _ -> [_]
            shift-left: T7."Drive2" -> [w458]
            shift-right: [w463] -> _
            shift-left: 0.0 ("y") -> [w464]
            tunnel: w453 -> [w462]
            tunnel: "Travel Distance (In) 6" -> [w461]
            tunnel: w449 -> [w460]
            tunnel: w448 -> [w459]
            stop <- w465 stop-if-true
            n232 = case shown="\"Drive2\"" w458 {
              tunnel: [FALSE FALSE FALSE FALSE FALSE FALSE FALSE FALSE FALSE FALSE TRUE] -> w465
              tunnel: w464 -> [w481 _ _ w542 _ _ _ _ w646 _ _]
              tunnel: [w480 0.0 0.0 w543 0.0 0.0 0.0 0.0 w647 0.0 0.0] -> w463
              tunnel: w462 -> [_ w506 _ _ _ _ w610 _ _ _ _]
              tunnel: w461 -> [_ w517 _ _ _ _ w621 _ _ _ _]
              tunnel: w460 -> [_ w495 w528 w552 w560 w576 w599 w632 w656 w664 w686]
              tunnel: w459 -> [_ w494 w527 w551 w559 w575 w598 w631 w655 w663 w685]
              tunnel: [w469 w491 _ w547 _ _ w595 _ w651 _ _] -> _
              frame "Init", Default {
                n233 = global read "GlobalRefnum.vi" "leftMotors"() -> (w473:string)
                n234 = global read "GlobalRefnum.vi" "rightMotors"() -> (w472:string)
                n235 = call <vilib>:"CTRE_Phoenix_MotorControl_RefNumRegistryGet.vi"("refnum name"=w473) -> ("error out"=w474:errorcluster, "PhoenixMotorControlDevRef"=w475:T9)  [unwired: 9 in]
                n236 = call <vilib>:"CTRE_Phoenix_MotorControl_RefNumRegistryGet.vi"("refnum name"=w472) -> ("error out"=w470:errorcluster, "PhoenixMotorControlDevRef"=w471:T9)  [unwired: 9 in]
                n237 = call <vilib>:"CTRE_Phoenix_MotorControl_SetSelectedSensorPosition.vi"("error in (no error)"=w474, "New Sensor Position"=0, "PhoenixMotorControlDevRef"=w475) -> ()  [unwired: 7 in, 2 out]
                n238 = call <vilib>:"CTRE_Phoenix_MotorControl_SetSelectedSensorPosition.vi"("error in (no error)"=w470, "New Sensor Position"=0, "PhoenixMotorControlDevRef"=w471) -> ()  [unwired: 7 in, 2 out]
                n239 = call-poly <vilib>:"NT Write Value.vi"("Numeric"=3.0, "Name"="/limelight/ledMode") -> ()  [unwired: 9 in, 1 out]
                n240 = Add(x=1.0, y=w481) -> (x+y=w480:dbl)
                n241 = Greater Or Equal?(x=w480, y=10.0) -> (x >= y?=w479:bool)
                n242 = Select(s=w479) -> (s? t:f=w469:dbl)  [unwired: 2 in]
              }
              frame "Drive" {
                n243 = Sign(1:w506) -> (0:w505:dbl)
                n244 = global write "Joystick_Buttons.vi" "right-Trigger"(TRUE ("left-ThumbR")) -> ()
                n245 = feedback #4() -> (w499:dbl)  [unwired: 1 in]
                n246 = Multiply(x=w505, y=w499) -> (x*y=w496:dbl)
                n247 = call-poly <vilib>:"WPI_RobotDriveArcadeDrive.vi"("error in (no error)"=w494, "X axis value"=w496, "RobotDriveDevRef"=w495) -> ()  [unwired: 6 in, 3 out]
                n248 = global read "Global Vars.vi" "RMPosition"() -> (w487:i32)
                n249 = global read "Global Vars.vi" "LMPosition"() -> (w493:i32)
                n250 = Absolute Value(x=w517) -> (abs(x)=w498:i32)
                n251 = Absolute Value(x=w487) -> (abs(x)=w484:i32)
                "Right Pos (In) 6" <- w484
                n252 = Greater?(x=w484, y=120000) -> (0:w485:bool)
                n253 = Absolute Value(x=w493) -> (abs(x)=w509:i32)
                "Left Pos (In) 6" <- w509
                n254 = Add(x=w509, y=w484) -> (x+y=w511:i32)
                n255 = Select(t="MaxDrive Slow 3", s=w485, f="MaxDrive Fast 4") -> (s? t:f=w488:dbl)
                n256 = Divide(x=w511, y=2.0) -> (x/y=w508:dbl)
                n257 = Absolute Value(x=w508) -> (abs(x)=w513:dbl)
                n258 = Subtract(x=w498, y=w508) -> (x-y=w516:dbl)
                n259 = Subtract(x=w498, y="DriveDeadband 6") -> (x-y=w503:dbl)
                n260 = Multiply(x=w516, y="DriveK 6") -> (x*y=w515:dbl)
                n261 = Negate(x=w488) -> (-x=w514:dbl)
                n262 = Subtract(x=w513, y=w503) -> (x-y=w502:dbl)
                n263 = Greater Than 0?(x=w502) -> (x > 0?=w501:bool)
                n264 = In Range and Coerce(upper limit=w488, x=w515, lower limit=w514) -> (coerced(x)=w497:dbl)  [unwired: 1 out]
                n265 = Greater Or Equal?(x=w509, y=w498) -> (x >= y?=w521:bool)
                n266 = Greater Or Equal?(x=w484, y=w498) -> (x >= y?=w520:bool)
                n267 = Or(x=w521, y=w520) -> (x .or. y?=w519:bool)
                n268 = Select(t=0.0, s=w501, f=w497) -> (s? t:f=w500:dbl)
                n269 = feedback-in #4(w500) -> ()
                n270 = Select(s=w519) -> (s? t:f=w491:dbl)  [unwired: 2 in]
              }
              frame "Pause1" {
                n271 = global read "GlobalRefnum.vi" "leftMotors"() -> (w534:string)
                n272 = global read "GlobalRefnum.vi" "rightMotors"() -> (w533:string)
                n273 = call <vilib>:"CTRE_Phoenix_MotorControl_RefNumRegistryGet.vi"("refnum name"=w534) -> ("error out"=w535:errorcluster, "PhoenixMotorControlDevRef"=w536:T9)  [unwired: 9 in]
                n274 = call <vilib>:"CTRE_Phoenix_MotorControl_RefNumRegistryGet.vi"("refnum name"=w533) -> ("error out"=w531:errorcluster, "PhoenixMotorControlDevRef"=w532:T9)  [unwired: 9 in]
                n275 = call <vilib>:"CTRE_Phoenix_MotorControl_SetSelectedSensorPosition.vi"("error in (no error)"=w535, "New Sensor Position"=0, "PhoenixMotorControlDevRef"=w536) -> ()  [unwired: 7 in, 2 out]
                n276 = call-poly <vilib>:"WPI_RobotDriveArcadeDrive.vi"("error in (no error)"=w527, "Y axis value"=0.0, "X axis value"=0.0, "RobotDriveDevRef"=w528) -> ()  [unwired: 5 in, 3 out]
                n277 = call <vilib>:"CTRE_Phoenix_MotorControl_SetSelectedSensorPosition.vi"("error in (no error)"=w531, "New Sensor Position"=0, "PhoenixMotorControlDevRef"=w532) -> ()  [unwired: 7 in, 2 out]
                n278 = call-poly <vilib>:"NT Write Value.vi"("Numeric"=0.0, "Name"="/limelight/camMode") -> ()  [unwired: 9 in, 1 out]
                n279 = Wait (ms)(milliseconds to wait=u32 50) -> ()  [unwired: 1 out]
              }
              frame "Aim" {
                n280 = global write "Joystick_Buttons.vi" "left-ThumbMain"(TRUE ("left-ThumbMain")) -> ()
                n281 = call "Limelight_Differential.vi"() -> ("DriveCommand"=w555:dbl, "SteerCommand"=w556:dbl)  [unwired: 8 in, 1 out]
                n282 = call-poly <vilib>:"NT Write Value.vi"("Numeric"=0.0, "Name"="/limelight/camMode") -> ()  [unwired: 9 in, 1 out]
                n283 = call-poly <vilib>:"NT Write Value.vi"("Numeric"=w556, "Name"="Aim Angle") -> ()  [unwired: 9 in, 1 out]
                n284 = call <vilib>:"WPI_RobotDriveArcadeDrive_Standard(NoSaturation).vi"("error in (no error)"=w551, "Y axis value"=w556, "X axis value"=w555, "RobotDriveDevRef"=w552) -> ("Motor Values"=w550:dbl[])  [unwired: 7 out]
                n285 = call-poly <vilib>:"NT Write Value.vi"("Numeric Array"=w550, "Name"="RobotDrive Motors") -> ()  [unwired: 9 in, 1 out]
                n286 = Add(x=1.0, y=w542) -> (x+y=w543:dbl)
                n287 = Greater Or Equal?(x=w543, y=100.0) -> (x >= y?=w544:bool)
                n288 = Select(s=w544) -> (s? t:f=w547:dbl)  [unwired: 2 in]
              }
              frame "Shoot" {
                n289 = call "Limelight_Differential.vi"() -> ("DriveCommand"=w564:dbl, "SteerCommand"=w565:dbl)  [unwired: 8 in, 1 out]
                n290 = call-poly <vilib>:"NT Write Value.vi"("Numeric"=w565, "Name"="Aim Angle") -> ()  [unwired: 9 in, 1 out]
                n291 = call <vilib>:"WPI_RobotDriveArcadeDrive_Standard(NoSaturation).vi"("error in (no error)"=w559, "Y axis value"=w565, "X axis value"=w564, "RobotDriveDevRef"=w560) -> ("Motor Values"=w562:dbl[])  [unwired: 7 out]
                n292 = call-poly <vilib>:"NT Write Value.vi"("Numeric Array"=w562, "Name"="RobotDrive Motors") -> ()  [unwired: 9 in, 1 out]
                n293 = global write "Joystick_Buttons.vi" "left-ThumbMain"(TRUE ("left-ThumbMain")) -> ()
                n294 = global write "Joystick_Buttons.vi" "left-Trigger"(TRUE ("left-ThumbR")) -> ()
                n295 = global write "Joystick_Buttons.vi" "right-Trigger"(TRUE ("left-ThumbMain")) -> ()
                n296 = global write "Joystick_Buttons.vi" "left-ThumbR"(TRUE ("left-ThumbMain")) -> ()
                n297 = Wait (ms)(milliseconds to wait=u32 5000) -> ()  [unwired: 1 out]
              }
              frame "Pause2" {
                n298 = global read "GlobalRefnum.vi" "leftMotors"() -> (w582:string)
                n299 = global read "GlobalRefnum.vi" "rightMotors"() -> (w581:string)
                n300 = call <vilib>:"CTRE_Phoenix_MotorControl_RefNumRegistryGet.vi"("refnum name"=w582) -> ("error out"=w583:errorcluster, "PhoenixMotorControlDevRef"=w584:T9)  [unwired: 9 in]
                n301 = call <vilib>:"CTRE_Phoenix_MotorControl_RefNumRegistryGet.vi"("refnum name"=w581) -> ("error out"=w579:errorcluster, "PhoenixMotorControlDevRef"=w580:T9)  [unwired: 9 in]
                n302 = call <vilib>:"CTRE_Phoenix_MotorControl_SetSelectedSensorPosition.vi"("error in (no error)"=w583, "New Sensor Position"=0, "PhoenixMotorControlDevRef"=w584) -> ()  [unwired: 7 in, 2 out]
                n303 = call-poly <vilib>:"WPI_RobotDriveArcadeDrive.vi"("error in (no error)"=w575, "Y axis value"=0.0, "X axis value"=0.0, "RobotDriveDevRef"=w576) -> ()  [unwired: 5 in, 3 out]
                n304 = call <vilib>:"CTRE_Phoenix_MotorControl_SetSelectedSensorPosition.vi"("error in (no error)"=w579, "New Sensor Position"=0, "PhoenixMotorControlDevRef"=w580) -> ()  [unwired: 7 in, 2 out]
                n305 = call-poly <vilib>:"NT Write Value.vi"("Numeric"=0.0, "Name"="/limelight/camMode") -> ()  [unwired: 9 in, 1 out]
                n306 = Wait (ms)(milliseconds to wait=u32 50) -> ()  [unwired: 1 out]
              }
              frame "Drive2" {
                n307 = Sign(1:w610) -> (0:w609:dbl)
                n308 = global write "Joystick_Buttons.vi" "right-Trigger"(TRUE ("left-ThumbR")) -> ()
                n309 = feedback #5() -> (w603:dbl)  [unwired: 1 in]
                n310 = Multiply(x=w609, y=w603) -> (x*y=w600:dbl)
                n311 = call-poly <vilib>:"WPI_RobotDriveArcadeDrive.vi"("error in (no error)"=w598, "X axis value"=w600, "RobotDriveDevRef"=w599) -> ()  [unwired: 6 in, 3 out]
                n312 = global read "Global Vars.vi" "RMPosition"() -> (w591:i32)
                n313 = global read "Global Vars.vi" "LMPosition"() -> (w597:i32)
                n314 = Absolute Value(x=w621) -> (abs(x)=w602:i32)
                n315 = Absolute Value(x=w591) -> (abs(x)=w588:i32)
                "Right Pos (In) 7" <- w588
                n316 = Greater?(x=w588, y=120000) -> (0:w589:bool)
                n317 = Absolute Value(x=w597) -> (abs(x)=w613:i32)
                "Left Pos (In) 7" <- w613
                n318 = Add(x=w613, y=w588) -> (x+y=w615:i32)
                n319 = Select(t="MaxDrive Slow 4", s=w589, f="MaxDrive Fast 5") -> (s? t:f=w592:dbl)
                n320 = Divide(x=w615, y=2.0) -> (x/y=w612:dbl)
                n321 = Absolute Value(x=w612) -> (abs(x)=w617:dbl)
                n322 = Subtract(x=w602, y=w612) -> (x-y=w620:dbl)
                n323 = Subtract(x=w602, y="DriveDeadband 7") -> (x-y=w607:dbl)
                n324 = Multiply(x=w620, y="DriveK 7") -> (x*y=w619:dbl)
                n325 = Negate(x=w592) -> (-x=w618:dbl)
                n326 = Subtract(x=w617, y=w607) -> (x-y=w606:dbl)
                n327 = Greater Than 0?(x=w606) -> (x > 0?=w605:bool)
                n328 = In Range and Coerce(upper limit=w592, x=w619, lower limit=w618) -> (coerced(x)=w601:dbl)  [unwired: 1 out]
                n329 = Greater Or Equal?(x=w613, y=w602) -> (x >= y?=w625:bool)
                n330 = Greater Or Equal?(x=w588, y=w602) -> (x >= y?=w624:bool)
                n331 = Or(x=w625, y=w624) -> (x .or. y?=w623:bool)
                n332 = Select(t=0.0, s=w605, f=w601) -> (s? t:f=w604:dbl)
                n333 = feedback-in #5(w604) -> ()
                n334 = Select(s=w623) -> (s? t:f=w595:dbl)  [unwired: 2 in]
              }
              frame "Pause3" {
                n335 = global read "GlobalRefnum.vi" "leftMotors"() -> (w638:string)
                n336 = global read "GlobalRefnum.vi" "rightMotors"() -> (w637:string)
                n337 = call <vilib>:"CTRE_Phoenix_MotorControl_RefNumRegistryGet.vi"("refnum name"=w638) -> ("error out"=w639:errorcluster, "PhoenixMotorControlDevRef"=w640:T9)  [unwired: 9 in]
                n338 = call <vilib>:"CTRE_Phoenix_MotorControl_RefNumRegistryGet.vi"("refnum name"=w637) -> ("error out"=w635:errorcluster, "PhoenixMotorControlDevRef"=w636:T9)  [unwired: 9 in]
                n339 = call <vilib>:"CTRE_Phoenix_MotorControl_SetSelectedSensorPosition.vi"("error in (no error)"=w639, "New Sensor Position"=0, "PhoenixMotorControlDevRef"=w640) -> ()  [unwired: 7 in, 2 out]
                n340 = call-poly <vilib>:"WPI_RobotDriveArcadeDrive.vi"("error in (no error)"=w631, "Y axis value"=0.0, "X axis value"=0.0, "RobotDriveDevRef"=w632) -> ()  [unwired: 5 in, 3 out]
                n341 = call <vilib>:"CTRE_Phoenix_MotorControl_SetSelectedSensorPosition.vi"("error in (no error)"=w635, "New Sensor Position"=0, "PhoenixMotorControlDevRef"=w636) -> ()  [unwired: 7 in, 2 out]
                n342 = call-poly <vilib>:"NT Write Value.vi"("Numeric"=0.0, "Name"="/limelight/camMode") -> ()  [unwired: 9 in, 1 out]
                n343 = Wait (ms)(milliseconds to wait=u32 50) -> ()  [unwired: 1 out]
              }
              frame "Pause3" {
                n344 = global write "Joystick_Buttons.vi" "left-ThumbMain"(TRUE ("left-ThumbMain")) -> ()
                n345 = call "Limelight_Differential.vi"() -> ("DriveCommand"=w659:dbl, "SteerCommand"=w660:dbl)  [unwired: 8 in, 1 out]
                n346 = call-poly <vilib>:"NT Write Value.vi"("Numeric"=0.0, "Name"="/limelight/camMode") -> ()  [unwired: 9 in, 1 out]
                n347 = call-poly <vilib>:"NT Write Value.vi"("Numeric"=w660, "Name"="Aim Angle") -> ()  [unwired: 9 in, 1 out]
                n348 = call <vilib>:"WPI_RobotDriveArcadeDrive_Standard(NoSaturation).vi"("error in (no error)"=w655, "Y axis value"=w660, "X axis value"=w659, "RobotDriveDevRef"=w656) -> ("Motor Values"=w654:dbl[])  [unwired: 7 out]
                n349 = call-poly <vilib>:"NT Write Value.vi"("Numeric Array"=w654, "Name"="RobotDrive Motors") -> ()  [unwired: 9 in, 1 out]
                n350 = Add(x=1.0, y=w646) -> (x+y=w647:dbl)
                n351 = Greater Or Equal?(x=w647, y=100.0) -> (x >= y?=w648:bool)
                n352 = Select(s=w648) -> (s? t:f=w651:dbl)  [unwired: 2 in]
              }
              frame "Shoot2" {
                n353 = call "Limelight_Differential.vi"() -> ("DriveCommand"=w668:dbl, "SteerCommand"=w669:dbl)  [unwired: 8 in, 1 out]
                n354 = call-poly <vilib>:"NT Write Value.vi"("Numeric"=w669, "Name"="Aim Angle") -> ()  [unwired: 9 in, 1 out]
                n355 = call <vilib>:"WPI_RobotDriveArcadeDrive_Standard(NoSaturation).vi"("error in (no error)"=w663, "Y axis value"=w669, "X axis value"=w668, "RobotDriveDevRef"=w664) -> ("Motor Values"=w666:dbl[])  [unwired: 7 out]
                n356 = call-poly <vilib>:"NT Write Value.vi"("Numeric Array"=w666, "Name"="RobotDrive Motors") -> ()  [unwired: 9 in, 1 out]
                n357 = global write "Joystick_Buttons.vi" "left-ThumbMain"(TRUE ("left-ThumbMain")) -> ()
                n358 = global write "Joystick_Buttons.vi" "left-Trigger"(TRUE ("left-ThumbR")) -> ()
                n359 = global write "Joystick_Buttons.vi" "right-Trigger"(TRUE ("left-ThumbMain")) -> ()
                n360 = global write "Joystick_Buttons.vi" "left-ThumbR"(TRUE ("left-ThumbMain")) -> ()
                n361 = Wait (ms)(milliseconds to wait=u32 5000) -> ()  [unwired: 1 out]
              }
              frame "End" {
                n362 = call <vilib>:"WPI_RobotDriveArcadeDrive_Standard(NoSaturation).vi"("error in (no error)"=w685, "Y axis value"=0.0, "X axis value"=0.0, "RobotDriveDevRef"=w686) -> ()  [unwired: 8 out]
                n363 = global write "Joystick_Buttons.vi" "right-Trigger"(FALSE ("left-ThumbR")) -> ()
                n364 = global write "Joystick_Buttons.vi" "left-ThumbMain"(FALSE ("left-ThumbMain")) -> ()
                n365 = global write "Joystick_Buttons.vi" "left-ThumbR"(FALSE ("left-ThumbMain")) -> ()
                n366 = global write "Joystick_Buttons.vi" "left-Trigger"(FALSE ("left-ThumbR")) -> ()
                n367 = call-poly <vilib>:"NT Write Value.vi"("Numeric"=1.0, "Name"="/limelight/camMode") -> ()  [unwired: 9 in, 1 out]
                n368 = Wait (ms)(milliseconds to wait=u32 50) -> ()  [unwired: 1 out]
              }
            }
            n369 = Wait (ms)(milliseconds to wait=u32 10) -> ()  [unwired: 1 out]
          }
        }
        frame Enabled {
        }
      }
    }
    frame "5BallTheirTrench" {
      w692 = 1.0
      n370 = Negate(x=w692) -> (-x=w693:dbl)
      n371 = global read "GlobalRefnum.vi" "twoMotorDrive"() -> (w691:string)
      n372 = Select(t=w693, s="Reverse? 5", f=w692) -> (s? t:f=w694:dbl)
      n373 = Wait (ms)(milliseconds to wait=u32 100) -> ()  [unwired: 1 out]
      n374 = call <vilib>:"WPI_RobotDriveRefNum Registry Get.vi"("refnum name"=w691) -> ("error out"=w689:errorcluster, "RobotDriveDevRef"=w690:T15)  [unwired: 9 in]
      n375 = while {
        shift-right: [w703] -> _
        shift-left: 0.0 ("y") -> [w704]
        tunnel: w694 -> [w702]
        tunnel: w690 -> [w701]
        tunnel: w689 -> [w700]
        shift-right: [w698] -> _
        shift-left: T8."Init" -> [w699]
        stop <- w705 stop-if-true
        n376 = case shown="\"End\"" w699 {
          tunnel: [FALSE FALSE FALSE FALSE FALSE FALSE FALSE FALSE TRUE] -> w705
          tunnel: w704 -> [w723 _ _ w788 _ _ w869 _ _]
          tunnel: [w722 0.0 0.0 w789 0.0 0.0 w870 0.0 0.0] -> w703
          tunnel: w702 -> [_ w751 _ _ _ w842 _ _ _]
          tunnel: w701 -> [_ w740 w773 w798 w807 w831 w861 w879 w904]
          tunnel: w700 -> [_ w739 w772 w797 w806 w830 w860 w878 w903]
          tunnel: [w711 w736 T8."Aim" w793 T8."Drive2" w827 w874 T8."End" T8."End"] -> w698
          frame "Init", Default {
            n377 = global read "GlobalRefnum.vi" "leftMotors"() -> (w715:string)
            n378 = global read "GlobalRefnum.vi" "rightMotors"() -> (w714:string)
            n379 = call <vilib>:"CTRE_Phoenix_MotorControl_RefNumRegistryGet.vi"("refnum name"=w715) -> ("error out"=w716:errorcluster, "PhoenixMotorControlDevRef"=w717:T9)  [unwired: 9 in]
            n380 = call <vilib>:"CTRE_Phoenix_MotorControl_RefNumRegistryGet.vi"("refnum name"=w714) -> ("error out"=w712:errorcluster, "PhoenixMotorControlDevRef"=w713:T9)  [unwired: 9 in]
            n381 = call <vilib>:"CTRE_Phoenix_MotorControl_SetSelectedSensorPosition.vi"("error in (no error)"=w716, "New Sensor Position"=0, "PhoenixMotorControlDevRef"=w717) -> ()  [unwired: 7 in, 2 out]
            n382 = call <vilib>:"CTRE_Phoenix_MotorControl_SetSelectedSensorPosition.vi"("error in (no error)"=w712, "New Sensor Position"=0, "PhoenixMotorControlDevRef"=w713) -> ()  [unwired: 7 in, 2 out]
            n383 = call-poly <vilib>:"NT Write Value.vi"("Numeric"=1.0, "Name"="/limelight/pipeline") -> ()  [unwired: 9 in, 1 out]
            n384 = Add(x=1.0, y=w723) -> (x+y=w722:dbl)
            n385 = Greater Or Equal?(x=w722, y=10.0) -> (x >= y?=w721:bool)
            n386 = Select(t=T8."Drive", s=w721, f=T8."Init") -> (s? t:f=w711:T8)
          }
          frame "Drive" {
            n387 = Sign(1:w751) -> (0:w750:dbl)
            n388 = global write "Joystick_Buttons.vi" "right-Trigger"(TRUE ("left-ThumbR")) -> ()
            n389 = feedback #6() -> (w744:dbl)  [unwired: 1 in]
            n390 = Multiply(x=w750, y=w744) -> (x*y=w741:dbl)
            n391 = call-poly <vilib>:"WPI_RobotDriveArcadeDrive.vi"("error in (no error)"=w739, "X axis value"=w741, "RobotDriveDevRef"=w740) -> ()  [unwired: 6 in, 3 out]
            n392 = global read "Global Vars.vi" "RMPosition"() -> (w732:i32)
            n393 = global read "Global Vars.vi" "LMPosition"() -> (w738:i32)
            n394 = Absolute Value(x="Travel Distance (In) 5") -> (abs(x)=w743:i32)
            n395 = Absolute Value(x=w732) -> (abs(x)=w729:i32)
            "Right Pos (In) 5" <- w729
            n396 = Greater?(x=w729, y=120000) -> (0:w730:bool)
            n397 = Absolute Value(x=w738) -> (abs(x)=w754:i32)
            "Left Pos (In) 5" <- w754
            n398 = Add(x=w754, y=w729) -> (x+y=w756:i32)
            n399 = Select(t="MaxDrive Slow 2", s=w730, f="MaxDrive Fast 2") -> (s? t:f=w733:dbl)
            n400 = Divide(x=w756, y=2.0) -> (x/y=w753:dbl)
            n401 = Absolute Value(x=w753) -> (abs(x)=w758:dbl)
            n402 = Subtract(x=w743, y=w753) -> (x-y=w761:dbl)
            n403 = Subtract(x=w743, y="DriveDeadband 4") -> (x-y=w748:dbl)
            n404 = Multiply(x=w761, y="DriveK 4") -> (x*y=w760:dbl)
            n405 = Negate(x=w733) -> (-x=w759:dbl)
            n406 = Subtract(x=w758, y=w748) -> (x-y=w747:dbl)
            n407 = Greater Than 0?(x=w747) -> (x > 0?=w746:bool)
            n408 = In Range and Coerce(upper limit=w733, x=w760, lower limit=w759) -> (coerced(x)=w742:dbl)  [unwired: 1 out]
            n409 = Greater Or Equal?(x=w754, y=w743) -> (x >= y?=w765:bool)
            n410 = Greater Or Equal?(x=w729, y=w743) -> (x >= y?=w764:bool)
            n411 = Or(x=w765, y=w764) -> (x .or. y?=w763:bool)
            n412 = Select(t=0.0, s=w746, f=w742) -> (s? t:f=w745:dbl)
            n413 = feedback-in #6(w745) -> ()
            n414 = Select(t=T8."Pause1", s=w763, f=T8."Drive") -> (s? t:f=w736:T8)
          }
          frame "Pause1" {
            n415 = global read "GlobalRefnum.vi" "leftMotors"() -> (w779:string)
            n416 = global read "GlobalRefnum.vi" "rightMotors"() -> (w778:string)
            n417 = call <vilib>:"CTRE_Phoenix_MotorControl_RefNumRegistryGet.vi"("refnum name"=w779) -> ("error out"=w780:errorcluster, "PhoenixMotorControlDevRef"=w781:T9)  [unwired: 9 in]
            n418 = call <vilib>:"CTRE_Phoenix_MotorControl_RefNumRegistryGet.vi"("refnum name"=w778) -> ("error out"=w776:errorcluster, "PhoenixMotorControlDevRef"=w777:T9)  [unwired: 9 in]
            n419 = call <vilib>:"CTRE_Phoenix_MotorControl_SetSelectedSensorPosition.vi"("error in (no error)"=w780, "New Sensor Position"=0, "PhoenixMotorControlDevRef"=w781) -> ()  [unwired: 7 in, 2 out]
            n420 = call-poly <vilib>:"WPI_RobotDriveArcadeDrive.vi"("error in (no error)"=w772, "Y axis value"=0.0, "X axis value"=0.0, "RobotDriveDevRef"=w773) -> ()  [unwired: 5 in, 3 out]
            n421 = call <vilib>:"CTRE_Phoenix_MotorControl_SetSelectedSensorPosition.vi"("error in (no error)"=w776, "New Sensor Position"=0, "PhoenixMotorControlDevRef"=w777) -> ()  [unwired: 7 in, 2 out]
            n422 = call-poly <vilib>:"NT Write Value.vi"("Numeric"=0.0, "Name"="/limelight/camMode") -> ()  [unwired: 9 in, 1 out]
            n423 = Wait (ms)(milliseconds to wait=u32 50) -> ()  [unwired: 1 out]
          }
          frame "Aim" {
            n424 = global write "Joystick_Buttons.vi" "left-ThumbMain"(FALSE ("left-ThumbMain")) -> ()
            n425 = call <vilib>:"WPI_RobotDriveArcadeDrive_Standard(NoSaturation).vi"("error in (no error)"=w797, "Y axis value"=0.5, "RobotDriveDevRef"=w798) -> ("Motor Values"=w796:dbl[])  [unwired: 1 in, 7 out]
            n426 = call-poly <vilib>:"NT Write Value.vi"("Numeric Array"=w796, "Name"="RobotDrive Motors") -> ()  [unwired: 9 in, 1 out]
            n427 = Add(x=1.0, y=w788) -> (x+y=w789:dbl)
            n428 = Greater Or Equal?(x=w789, y=150.0) -> (x >= y?=w790:bool)
            n429 = Select(t=T8."Pause2", s=w790, f=T8."Aim") -> (s? t:f=w793:T8)
          }
          frame "Pause2" {
            n430 = global read "GlobalRefnum.vi" "leftMotors"() -> (w813:string)
            n431 = global read "GlobalRefnum.vi" "rightMotors"() -> (w812:string)
            n432 = call <vilib>:"CTRE_Phoenix_MotorControl_RefNumRegistryGet.vi"("refnum name"=w813) -> ("error out"=w814:errorcluster, "PhoenixMotorControlDevRef"=w815:T9)  [unwired: 9 in]
            n433 = call <vilib>:"CTRE_Phoenix_MotorControl_RefNumRegistryGet.vi"("refnum name"=w812) -> ("error out"=w810:errorcluster, "PhoenixMotorControlDevRef"=w811:T9)  [unwired: 9 in]
            n434 = call <vilib>:"CTRE_Phoenix_MotorControl_SetSelectedSensorPosition.vi"("error in (no error)"=w814, "New Sensor Position"=0, "PhoenixMotorControlDevRef"=w815) -> ()  [unwired: 7 in, 2 out]
            n435 = call-poly <vilib>:"WPI_RobotDriveArcadeDrive.vi"("error in (no error)"=w806, "Y axis value"=0.0, "X axis value"=0.0, "RobotDriveDevRef"=w807) -> ()  [unwired: 5 in, 3 out]
            n436 = call <vilib>:"CTRE_Phoenix_MotorControl_SetSelectedSensorPosition.vi"("error in (no error)"=w810, "New Sensor Position"=0, "PhoenixMotorControlDevRef"=w811) -> ()  [unwired: 7 in, 2 out]
            n437 = global write "Joystick_Buttons.vi" "left-ThumbMain"(FALSE ("left-ThumbMain")) -> ()
            n438 = call-poly <vilib>:"NT Write Value.vi"("Numeric"=0.0, "Name"="/limelight/camMode") -> ()  [unwired: 9 in, 1 out]
            n439 = Wait (ms)(milliseconds to wait=u32 50) -> ()  [unwired: 1 out]
          }
          frame "Drive2" {
            n440 = Sign(1:w842) -> (0:w841:dbl)
            n441 = global write "Joystick_Buttons.vi" "left-ThumbMain"(FALSE ("left-ThumbMain")) -> ()
            n442 = global write "Joystick_Buttons.vi" "right-Trigger"(TRUE ("left-ThumbR")) -> ()
            n443 = feedback #7() -> (w835:dbl)  [unwired: 1 in]
            n444 = Multiply(x=w841, y=w835) -> (x*y=w832:dbl)
            n445 = Negate(x=w832) -> (-x=w823:dbl)
            n446 = call-poly <vilib>:"WPI_RobotDriveArcadeDrive.vi"("error in (no error)"=w830, "X axis value"=w823, "RobotDriveDevRef"=w831) -> ()  [unwired: 6 in, 3 out]
            n447 = global read "Global Vars.vi" "RMPosition"() -> (w826:i32)
            n448 = global read "Global Vars.vi" "LMPosition"() -> (w829:i32)
            n449 = Absolute Value(x="Travel Distance 2") -> (abs(x)=w834:i32)
            n450 = Absolute Value(x=w826) -> (abs(x)=w825:i32)
            n451 = Absolute Value(x=w829) -> (abs(x)=w845:i32)
            n452 = Add(x=w845, y=w825) -> (x+y=w847:i32)
            n453 = Divide(x=w847, y=2.0) -> (x/y=w844:dbl)
            n454 = Absolute Value(x=w844) -> (abs(x)=w849:dbl)
            n455 = Subtract(x=w834, y=w844) -> (x-y=w852:dbl)
            n456 = Subtract(x=w834, y="DriveDeadband 5") -> (x-y=w839:dbl)
            n457 = Multiply(x=w852, y="DriveK 5") -> (x*y=w851:dbl)
            n458 = Negate(x="MaxDrive Fast 3") -> (-x=w850:dbl)
            n459 = Subtract(x=w849, y=w839) -> (x-y=w838:dbl)
            n460 = Greater Than 0?(x=w838) -> (x > 0?=w837:bool)
            n461 = In Range and Coerce(upper limit="MaxDrive Fast 3", x=w851, lower limit=w850) -> (coerced(x)=w833:dbl)  [unwired: 1 out]
            n462 = Greater Or Equal?(x=w845, y=w834) -> (x >= y?=w856:bool)
            n463 = Greater Or Equal?(x=w825, y=w834) -> (x >= y?=w855:bool)
            n464 = Or(x=w856, y=w855) -> (x .or. y?=w854:bool)
            n465 = Select(t=0.0, s=w837, f=w833) -> (s? t:f=w836:dbl)
            n466 = feedback-in #7(w836) -> ()
            n467 = Select(t=T8."Aim2", s=w854, f=T8."Drive2") -> (s? t:f=w827:T8)
          }
          frame "Aim2" {
            n468 = global write "Joystick_Buttons.vi" "left-ThumbMain"(TRUE ("left-ThumbMain")) -> ()
            n469 = call "Limelight_Differential.vi"() -> ("DriveCommand"=w865:dbl, "SteerCommand"=w866:dbl)  [unwired: 8 in, 1 out]
            n470 = call-poly <vilib>:"NT Write Value.vi"("Numeric"=w866, "Name"="Aim Angle") -> ()  [unwired: 9 in, 1 out]
            n471 = call <vilib>:"WPI_RobotDriveArcadeDrive_Standard(NoSaturation).vi"("error in (no error)"=w860, "Y axis value"=w866, "X axis value"=w865, "RobotDriveDevRef"=w861) -> ("Motor Values"=w863:dbl[])  [unwired: 7 out]
            n472 = call-poly <vilib>:"NT Write Value.vi"("Numeric Array"=w863, "Name"="RobotDrive Motors") -> ()  [unwired: 9 in, 1 out]
            n473 = Add(x=1.0, y=w869) -> (x+y=w870:dbl)
            n474 = call-poly <vilib>:"NT Write Value.vi"("Numeric"=0.0, "Name"="/limelight/camMode") -> ()  [unwired: 9 in, 1 out]
            n475 = Greater Or Equal?(x=w870, y=100.0) -> (x >= y?=w871:bool)
            n476 = Select(t=T8."Shoot", s=w871, f=T8."Aim2") -> (s? t:f=w874:T8)
          }
          frame "Shoot" {
            n477 = call "Limelight_Differential.vi"() -> ("DriveCommand"=w883:dbl, "SteerCommand"=w884:dbl)  [unwired: 8 in, 1 out]
            n478 = call-poly <vilib>:"NT Write Value.vi"("Numeric"=w884, "Name"="Aim Angle") -> ()  [unwired: 9 in, 1 out]
            n479 = call <vilib>:"WPI_RobotDriveArcadeDrive_Standard(NoSaturation).vi"("error in (no error)"=w878, "Y axis value"=w884, "X axis value"=w883, "RobotDriveDevRef"=w879) -> ("Motor Values"=w881:dbl[])  [unwired: 7 out]
            n480 = call-poly <vilib>:"NT Write Value.vi"("Numeric Array"=w881, "Name"="RobotDrive Motors") -> ()  [unwired: 9 in, 1 out]
            n481 = global write "Joystick_Buttons.vi" "left-ThumbMain"(TRUE ("left-ThumbMain")) -> ()
            n482 = global write "Joystick_Buttons.vi" "left-Trigger"(TRUE ("left-ThumbR")) -> ()
            n483 = Wait (ms)(milliseconds to wait=u32 5000) -> ()  [unwired: 1 out]
          }
          frame "End" {
            n484 = call <vilib>:"WPI_RobotDriveArcadeDrive_Standard(NoSaturation).vi"("error in (no error)"=w903, "Y axis value"=0.0, "X axis value"=0.0, "RobotDriveDevRef"=w904) -> ()  [unwired: 8 out]
            n485 = global write "Joystick_Buttons.vi" "right-Trigger"(FALSE ("left-ThumbR")) -> ()
            n486 = global write "Joystick_Buttons.vi" "left-ThumbMain"(FALSE ("left-ThumbMain")) -> ()
            n487 = global write "Joystick_Buttons.vi" "left-ThumbR"(FALSE ("left-ThumbMain")) -> ()
            n488 = global write "Joystick_Buttons.vi" "left-Trigger"(FALSE ("left-ThumbR")) -> ()
            n489 = call-poly <vilib>:"NT Write Value.vi"("Numeric"=1.0, "Name"="/limelight/camMode") -> ()  [unwired: 9 in, 1 out]
            n490 = Wait (ms)(milliseconds to wait=u32 50) -> ()  [unwired: 1 out]
            n491 = call-poly <vilib>:"NT Write Value.vi"("Numeric"=0.0, "Name"="/limelight/pipeline") -> ()  [unwired: 9 in, 1 out]
          }
        }
        n492 = Wait (ms)(milliseconds to wait=u32 10) -> ()  [unwired: 1 out]
      }
    }
    frame "Alternative 1" {
      # "stand still"
      # "This sample code describes robot movements in an array. You can extend it to control other motors\non your robot. You can also use file I/O to move the data to a text file."
      n493 = call <vilib>:"WPI_RobotDriveRefNum Registry Get.vi"("refnum name"="Left and Right Motors") -> ("RobotDriveDevRef"=w912:T15)  [unwired: 1 in, 9 out]
      n494 = for {
        shift-right: [w920] -> w907
        shift-left: w912 -> [w921]
        tunnel: "Array of robot movements" -> [w916] mode=indexing
        n495 = Unbundle By Name(w916) -> ("X Joystick Value"=w919:dbl, "Y Joystick Value"=w918:dbl, "Delay (sec)"=w917:dbl)  [unwired: 1 out]
        n496 = call-poly <vilib>:"WPI_RobotDriveArcadeDrive.vi"("Y axis value"=w918, "X axis value"=w919, "RobotDriveDevRef"=w921) -> ("Motor Values"=w914:dbl[], "RobotDriveDevRef"=w922:T15)  [unwired: 1 in, 6 out]
        n497 = call-poly <vilib>:"NT Write Value.vi"("Numeric Array"=w914, "Name"="RobotDrive Motors") -> ()  [unwired: 9 in, 1 out]
        n498 = call <vilib>:"WPI_RobotDriveDelayAndUpdateSafety.vi"("Delay (s)"=w917, "RobotDriveDevRef"=w922) -> ("RobotDriveDevRef 2"=w920:T15)  [unwired: 8 in, 1 out]
        "Current Movement, for debugging" <- w916
      }
      n499 = call-poly <vilib>:"WPI_RobotDriveArcadeDrive.vi"("Y axis value"=0.0 ("X axis value"), "X axis value"=0.0, "RobotDriveDevRef"=w907) -> ("Motor Values"=w910:dbl[])  [unwired: 1 in, 7 out]
      n500 = call-poly <vilib>:"NT Write Value.vi"("Numeric Array"=w910, "Name"="RobotDrive Motors") -> ()  [unwired: 9 in, 1 out]
    }
    frame "Alternative 2" {
      w924 = "RobotDrive Motors" ("Name")
      # "This is some simple sample code to drive your robot curving one direction and then the other."
      # "stand still"
      # "other way for 0.5 second"
      # "turn for 1 second"
      n501 = call <vilib>:"WPI_RobotDriveRefNum Registry Get.vi"("refnum name"="Left and Right Motors") -> ("RobotDriveDevRef"=w940:T15)  [unwired: 1 in, 9 out]
      n502 = call-poly <vilib>:"WPI_RobotDriveArcadeDrive.vi"("Y axis value"=0.5 ("X axis value"), "X axis value"=-0.25, "RobotDriveDevRef"=w940) -> ("Motor Values"=w923:dbl[], "RobotDriveDevRef"=w933:T15)  [unwired: 1 in, 6 out]
      n503 = call-poly <vilib>:"NT Write Value.vi"("Numeric Array"=w923, "Name"=w924) -> ()  [unwired: 9 in, 1 out]
      n504 = call <vilib>:"WPI_RobotDriveDelayAndUpdateSafety.vi"("Delay (s)"=1.0, "RobotDriveDevRef"=w933) -> ("RobotDriveDevRef 2"=w934:T15)  [unwired: 8 in, 1 out]
      n505 = call-poly <vilib>:"WPI_RobotDriveArcadeDrive.vi"("Y axis value"=-0.25 ("X axis value"), "X axis value"=0.5, "RobotDriveDevRef"=w934) -> ("Motor Values"=w925:dbl[], "RobotDriveDevRef"=w935:T15)  [unwired: 1 in, 6 out]
      n506 = call-poly <vilib>:"NT Write Value.vi"("Numeric Array"=w925, "Name"=w924) -> ()  [unwired: 9 in, 1 out]
      n507 = call <vilib>:"WPI_RobotDriveDelayAndUpdateSafety.vi"("Delay (s)"=0.5, "RobotDriveDevRef"=w935) -> ("RobotDriveDevRef 2"=w936:T15)  [unwired: 8 in, 1 out]
      n508 = call-poly <vilib>:"WPI_RobotDriveArcadeDrive.vi"("Y axis value"=0.0 ("X axis value"), "X axis value"=0.0, "RobotDriveDevRef"=w936) -> ("Motor Values"=w926:dbl[])  [unwired: 1 in, 7 out]
      n509 = call-poly <vilib>:"NT Write Value.vi"("Numeric Array"=w926, "Name"=w924) -> ()  [unwired: 9 in, 1 out]
    }
    frame "Your Turn" {
      n510 = global read "GlobalRefnum.vi" "twoMotorDrive"() -> (w946:string)
      n511 = call <vilib>:"WPI_RobotDriveRefNum Registry Get.vi"("refnum name"=w946) -> ("error out"=w948:errorcluster, "RobotDriveDevRef"=w947:T15)  [unwired: 9 in]
      n512 = call-poly <vilib>:"WPI_RobotDriveArcadeDrive.vi"("error in (no error)"=w948, "Y axis value"=0.5, "X axis value"=0.5, "RobotDriveDevRef"=w947) -> ("error out"=w944:errorcluster, "RobotDriveDevRef"=w945:T15)  [unwired: 5 in, 1 out]
      n513 = call <vilib>:"WPI_RobotDriveDelayAndUpdateSafety.vi"("error in (no error)"=w944, "Delay (s)"=2.0, "RobotDriveDevRef"=w945) -> ()  [unwired: 7 in, 2 out]
    }
  }
